vi "3_AdvancedDemo_MHT3.vi"() -> ()   [LabVIEW 2019]
uses:
  <userlib>/MultiHarp150/demos/Types/MH_InputChannel.ctl
  <userlib>/MultiHarp150/demos/Types/MH_UIThread_Cmds.ctl
  <userlib>/MultiHarp150/demos/Types/MH_UIThread_Data.ctl
  <userlib>/MultiHarp150/demos/_lib/PQ/MultiHarp/MH_InitInfo.ctl
  <userlib>/MultiHarp150/UIThread/MH_SetInpChanData.ctl
  <userlib>/MultiHarp150/UIThread/MH_SetInpChanCmds.ctl
  <userlib>/MultiHarp150/demos/Types/MH_DataProcThread_QData.ctl
  <userlib>/MultiHarp150/demos/Types/MH_DataProcThread_QCmds.ctl
  <userlib>/MultiHarp150/demos/Types/MH_VisThread_QData.ctl
  <userlib>/MultiHarp150/demos/Types/MH_VisThread_QCmds.ctl
  <userlib>/MultiHarp150/demos/Types/MH_VisThread_Data.ctl
  <userlib>/MultiHarp150/MH_RefSource.ctl
  <userlib>/MultiHarp150/MH_MeasMode.ctl
  <vilib>/Utility/error.llb/DialogType.ctl
  <userlib>/MultiHarp150/MH_LibVersion_global.vi
  <userlib>/MultiHarp150/MH_DllPath_global.vi
panel:
  in  "Settings":bool=TRUE
  in  "Run continuously":bool caption="Conti."
  in  "Start":bool
  in  "Scale":bool
  out "CountRates":i32[](graph)
  in  "AllChannels":T1={"Enable"=TRUE, "Offset"=0, "Level"=-100, "Edge"=0, "DeadTime"=1000, "UseDeadTime"=FALSE, "SetEnableAllChan"=TRUE, "SetEdgeAllChan"=TRUE, "SetLevelAllChan"=TRUE, "SetOffsetAllChan"=TRUE, "SetUseDTAllChan"=TRUE, "SetDeadTAllChan"=TRUE} {"DeadTime" min=800 max=160000 step=1; "Edge" items=["falling", "rising"]; "Offset" min=-100000 max=100000 step=5; "Level" min=-1200 max=1200 step=1}
  in  "HistoAcqTime":dbl=1.0 caption="Hist.Int.Time  s" min=0.1 max=360000.0 step=0.1
  in  "AcqTime":i32=360000000 caption="T3Acqu.       ms" min=1 max=360000 step=1
  in  "Binning":i32(ring) caption="Resol.            ps" items=["5", "10", "20", "40", "80", "160", "320", "640", "1280", "2560", "5120", "10240", "20480", "40960", "81920", "163840", "327680", "655360", "1310720", "2621440", "5242880", "10485760", "20971520", "41943040"]
  in  "HistoOffset":i32 caption="Offset            ns" min=0 max=100000000 step=1
  out "DeltaT":dbl=2.0479769602591973 caption="T.Tr.Resol.   ms" format="%.2f"
  in  "BitShift":i32=15 min=0 max=32 step=1
  in  "OvlLevel":u32=4294967295 caption="Ovl.Level" min=1024 max=65536 step=1024
  in  "StopOvl.":bool=TRUE
  out "TTraceGraph":T2(graph)={49.38852226226715, "Resolution"=0.00655367864414373, "Histogram"=[]}
  out "HistoGraph":cluster{dbl, "Resol":dbl, "Histos":u32[][]}(graph)={0.0, "Resol"=0.08, "Histos"=[]}
  in  "SyncDeadTime":i32=1000 caption="Dead T.   ps" min=800 max=160000 step=1
  in  "UseDeadTime":bool caption="Use DT."
  in  "SyncEdge":i32(ring) caption="Edge" items=["falling", "rising"]
  in  "SyncDivider":i32(ring) caption="Divider" items=["1", "2", "4", "8", "16"]
  in  "SyncOffset":i32 caption="Offset      ps" min=-100000 max=100000 step=5
  in  "SyncLevel":i32=-100 caption="Level      mV" min=-1200 max=1200 step=1
  in  "Channels":T3[](array[typedef])=[{"Name"="Inp.Chan 1", "Enable"=TRUE, "Edge"=0, "Level"=-100, "Offset"=0, "UseDeadTime"=FALSE, "DeadTime"=1000}, {"Name"="Inp.Chan 2", "Enable"=TRUE, "Edge"=0, "Level"=-100, "Offset"=0, "UseDeadTime"=FALSE, "DeadTime"=1000}, {"Name"="Inp.Chan 3", "Enable"=TRUE, "Edge"=0, "Level"=-100, "Offset"=0, "UseDeadTime"=FALSE, "DeadTime"=1000}, {"Name"="Inp.Chan 4", "Enable"=TRUE, "Edge"=0, "Level"=-100, "Offset"=0, "UseDeadTime"=FALSE, "DeadTime"=1000}, {"Name"="Inp.Chan 5", "Enable"=TRUE, "Edge"=0, "Level"=-100, "Offset"=0, "UseDeadTime"=FALSE, "DeadTime"=1000}, {"Name"="Inp.Chan 6", "Enable"=TRUE, "Edge"=0, "Level"=-100, "Offset"=0, "UseDeadTime"=FALSE, "DeadTime"=1000}, {"Name"="Inp.Chan 7", "Enable"=TRUE, "Edge"=0, "Level"=-100, "Offset"=0, "UseDeadTime"=FALSE, "DeadTime"=1000}, {"Name"="Inp.Chan 8", "Enable"=TRUE, "Edge"=0, "Level"=-100, "Offset"=0, "UseDeadTime"=FALSE, "DeadTime"=1000}, {"Name"="Inp.Chan 9", "Enable"=TRUE, "Edge"=0, "Level"=-100, "Offset"=0, "UseDeadTime"=FALSE, "DeadTime"=1000}, {"Name"="Inp.Chan 10", "Enable"=TRUE, "Edge"=0, "Level"=-100, "Offset"=0, "UseDeadTime"=FALSE, "DeadTime"=1000}, {"Name"="Inp.Chan 11", "Enable"=TRUE, "Edge"=0, "Level"=-100, "Offset"=0, "UseDeadTime"=FALSE, "DeadTime"=1000}, {"Name"="Inp.Chan 12", "Enable"=TRUE, "Edge"=0, "Level"=-100, "Offset"=0, "UseDeadTime"=FALSE, "DeadTime"=1000}, {"Name"="Inp.Chan 13", "Enable"=TRUE, "Edge"=0, "Level"=-100, "Offset"=0, "UseDeadTime"=FALSE, "DeadTime"=1000}, {"Name"="Inp.Chan 14", "Enable"=TRUE, "Edge"=0, "Level"=-100, "Offset"=0, "UseDeadTime"=FALSE, "DeadTime"=1000}, {"Name"="Inp.Chan 15", "Enable"=TRUE, "Edge"=0, "Level"=-100, "Offset"=0, "UseDeadTime"=FALSE, "DeadTime"=1000}, {"Name"="Inp.Chan 16", "Enable"=TRUE, "Edge"=0, "Level"=-100, "Offset"=0, "UseDeadTime"=FALSE, "DeadTime"=1000}, {"Name"="Inp.Chan 17", "Enable"=TRUE, "Edge"=0, "Level"=-100, "Offset"=0, "UseDeadTime"=FALSE, "DeadTime"=1000}, {"Name"="Inp.Chan 18", "Enable"=TRUE, "Edge"=0, "Level"=-100, "Offset"=0, "UseDeadTime"=FALSE, "DeadTime"=1000}, {"Name"="Inp.Chan 19", "Enable"=TRUE, "Edge"=0, "Level"=-100, "Offset"=0, "UseDeadTime"=FALSE, "DeadTime"=1000}, {"Name"="Inp.Chan 20", "Enable"=TRUE, "Edge"=0, "Level"=-100, "Offset"=0, "UseDeadTime"=FALSE, "DeadTime"=1000}, {"Name"="Inp.Chan 21", "Enable"=TRUE, "Edge"=0, "Level"=-100, "Offset"=0, "UseDeadTime"=FALSE, "DeadTime"=1000}, {"Name"="Inp.Chan 22", "Enable"=TRUE, "Edge"=0, "Level"=-100, "Offset"=0, "UseDeadTime"=FALSE, "DeadTime"=1000}, {"Name"="Inp.Chan 23", "Enable"=TRUE, "Edge"=0, "Level"=-100, "Offset"=0, "UseDeadTime"=FALSE, "DeadTime"=1000}, {"Name"="Inp.Chan 24", "Enable"=TRUE, "Edge"=0, "Level"=-100, "Offset"=0, "UseDeadTime"=FALSE, "DeadTime"=1000}, {"Name"="Inp.Chan 25", "Enable"=TRUE, "Edge"=0, "Level"=-100, "Offset"=0, "UseDeadTime"=FALSE, "DeadTime"=1000}, {"Name"="Inp.Chan 26", "Enable"=TRUE, "Edge"=0, "Level"=-100, "Offset"=0, "UseDeadTime"=FALSE, "DeadTime"=1000}, {"Name"="Inp.Chan 27", "Enable"=TRUE, "Edge"=0, "Level"=-100, "Offset"=0, "UseDeadTime"=FALSE, "DeadTime"=1000}, {"Name"="Inp.Chan 28", "Enable"=TRUE, "Edge"=0, "Level"=-100, "Offset"=0, "UseDeadTime"=FALSE, "DeadTime"=1000}, {"Name"="Inp.Chan 29", "Enable"=TRUE, "Edge"=0, "Level"=-100, "Offset"=0, "UseDeadTime"=FALSE, "DeadTime"=1000}, {"Name"="Inp.Chan 30", "Enable"=TRUE, "Edge"=0, "Level"=-100, "Offset"=0, "UseDeadTime"=FALSE, "DeadTime"=1000}, {"Name"="Inp.Chan 31", "Enable"=TRUE, "Edge"=0, "Level"=-100, "Offset"=0, "UseDeadTime"=FALSE, "DeadTime"=1000}, {"Name"="Inp.Chan 32", "Enable"=TRUE, "Edge"=0, "Level"=-100, "Offset"=0, "UseDeadTime"=FALSE, "DeadTime"=1000}, {"Name"="Inp.Chan 33", "Enable"=TRUE, "Edge"=0, "Level"=-100, "Offset"=0, "UseDeadTime"=FALSE, "DeadTime"=1000}, {"Name"="Inp.Chan 34", "Enable"=TRUE, "Edge"=0, "Level"=-100, "Offset"=0, "UseDeadTime"=FALSE, "DeadTime"=1000}, {"Name"="Inp.Chan 35", "Enable"=TRUE, "Edge"=0, "Level"=-100, "Offset"=0, "UseDeadTime"=FALSE, "DeadTime"=1000}, {"Name"="Inp.Chan 36", "Enable"=TRUE, "Edge"=0, "Level"=-100, "Offset"=0, "UseDeadTime"=FALSE, "DeadTime"=1000}, {"Name"="Inp.Chan 37", "Enable"=TRUE, "Edge"=0, "Level"=-100, "Offset"=0, "UseDeadTime"=FALSE, "DeadTime"=1000}, {"Name"="Inp.Chan 38", "Enable"=TRUE, "Edge"=0, "Level"=-100, "Offset"=0, "UseDeadTime"=FALSE, "DeadTime"=1000}, {"Name"="Inp.Chan 39", "Enable"=TRUE, "Edge"=0, "Level"=-100, "Offset"=0, "UseDeadTime"=FALSE, "DeadTime"=1000}, {"Name"="Inp.Chan 40", "Enable"=TRUE, "Edge"=0, "Level"=-100, "Offset"=0, "UseDeadTime"=FALSE, "DeadTime"=1000}, {"Name"="Inp.Chan 41", "Enable"=TRUE, "Edge"=0, "Level"=-100, "Offset"=0, "UseDeadTime"=FALSE, "DeadTime"=1000}, {"Name"="Inp.Chan 42", "Enable"=TRUE, "Edge"=0, "Level"=-100, "Offset"=0, "UseDeadTime"=FALSE, "DeadTime"=1000}, {"Name"="Inp.Chan 43", "Enable"=TRUE, "Edge"=0, "Level"=-100, "Offset"=0, "UseDeadTime"=FALSE, "DeadTime"=1000}, {"Name"="Inp.Chan 44", "Enable"=TRUE, "Edge"=0, "Level"=-100, "Offset"=0, "UseDeadTime"=FALSE, "DeadTime"=1000}, {"Name"="Inp.Chan 45", "Enable"=TRUE, "Edge"=0, "Level"=-100, "Offset"=0, "UseDeadTime"=FALSE, "DeadTime"=1000}, {"Name"="Inp.Chan 46", "Enable"=TRUE, "Edge"=0, "Level"=-100, "Offset"=0, "UseDeadTime"=FALSE, "DeadTime"=1000}, {"Name"="Inp.Chan 47", "Enable"=TRUE, "Edge"=0, "Level"=-100, "Offset"=0, "UseDeadTime"=FALSE, "DeadTime"=1000}, {"Name"="Inp.Chan 48", "Enable"=TRUE, "Edge"=0, "Level"=-100, "Offset"=0, "UseDeadTime"=FALSE, "DeadTime"=1000}, {"Name"="Inp.Chan 49", "Enable"=TRUE, "Edge"=0, "Level"=-100, "Offset"=0, "UseDeadTime"=FALSE, "DeadTime"=1000}, {"Name"="Inp.Chan 50", "Enable"=TRUE, "Edge"=0, "Level"=-100, "Offset"=0, "UseDeadTime"=FALSE, "DeadTime"=1000}, {"Name"="Inp.Chan 51", "Enable"=TRUE, "Edge"=0, "Level"=-100, "Offset"=0, "UseDeadTime"=FALSE, "DeadTime"=1000}, {"Name"="Inp.Chan 52", "Enable"=TRUE, "Edge"=0, "Level"=-100, "Offset"=0, "UseDeadTime"=FALSE, "DeadTime"=1000}, {"Name"="Inp.Chan 53", "Enable"=TRUE, "Edge"=0, "Level"=-100, "Offset"=0, "UseDeadTime"=FALSE, "DeadTime"=1000}, {"Name"="Inp.Chan 54", "Enable"=TRUE, "Edge"=0, "Level"=-100, "Offset"=0, "UseDeadTime"=FALSE, "DeadTime"=1000}, {"Name"="Inp.Chan 55", "Enable"=TRUE, "Edge"=0, "Level"=-100, "Offset"=0, "UseDeadTime"=FALSE, "DeadTime"=1000}, {"Name"="Inp.Chan 56", "Enable"=TRUE, "Edge"=0, "Level"=-100, "Offset"=0, "UseDeadTime"=FALSE, "DeadTime"=1000}, {"Name"="Inp.Chan 57", "Enable"=TRUE, "Edge"=0, "Level"=-100, "Offset"=0, "UseDeadTime"=FALSE, "DeadTime"=1000}, {"Name"="Inp.Chan 58", "Enable"=TRUE, "Edge"=0, "Level"=-100, "Offset"=0, "UseDeadTime"=FALSE, "DeadTime"=1000}, {"Name"="Inp.Chan 59", "Enable"=TRUE, "Edge"=0, "Level"=-100, "Offset"=0, "UseDeadTime"=FALSE, "DeadTime"=1000}, {"Name"="Inp.Chan 60", "Enable"=TRUE, "Edge"=0, "Level"=-100, "Offset"=0, "UseDeadTime"=FALSE, "DeadTime"=1000}, {"Name"="Inp.Chan 61", "Enable"=TRUE, "Edge"=0, "Level"=-100, "Offset"=0, "UseDeadTime"=FALSE, "DeadTime"=1000}, {"Name"="Inp.Chan 62", "Enable"=TRUE, "Edge"=0, "Level"=-100, "Offset"=0, "UseDeadTime"=FALSE, "DeadTime"=1000}, {"Name"="Inp.Chan 63", "Enable"=TRUE, "Edge"=0, "Level"=-100, "Offset"=0, "UseDeadTime"=FALSE, "DeadTime"=1000}, {"Name"="Inp.Chan 64", "Enable"=TRUE, "Edge"=0, "Level"=-100, "Offset"=0, "UseDeadTime"=FALSE, "DeadTime"=1000}] {"DeadTime" min=800 max=160000 step=1; "Edge" items=["falling", "rising"]; "Offset" min=-100000 max=100000 step=5; "Level" min=-1200 max=1200 step=1}
  out "SyncRate":string="Sync Rate: 16000190 cps\n"
  out "OverRun":bool caption="Overrun:"
  out "Status":string="Elements in Q: 0"
  # "All Channels"
  # "Acquisition"
  # "Sync"
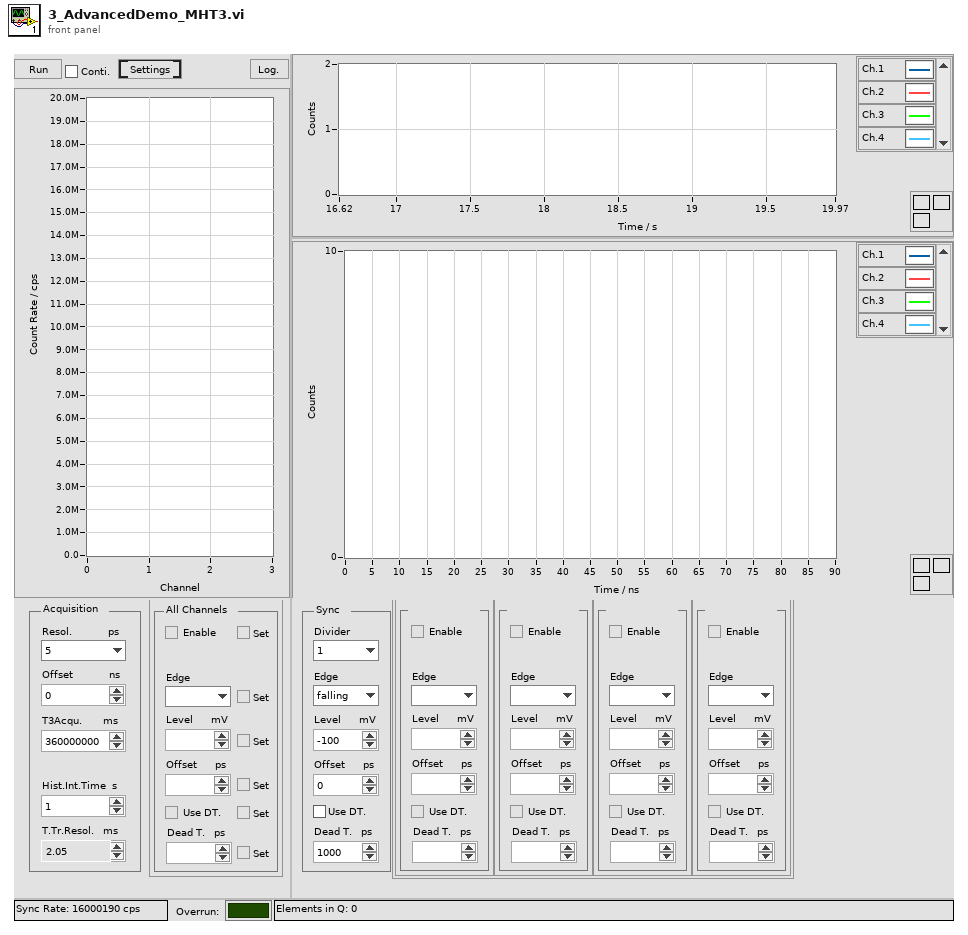
[diagram p1: front panel]
types:
  T1 = cluster{"Enable":bool, "Offset":i32, "Level":i32, "Edge":i32, "DeadTime":i32, "UseDeadTime":bool, "SetEnableAllChan":bool, "SetEdgeAllChan":bool, "SetLevelAllChan":bool, "SetOffsetAllChan":bool, "SetUseDTAllChan":bool, "SetDeadTAllChan":bool}
  T2 = cluster{dbl, "Resolution":dbl, "Histogram":u32[][]}
  T3 = typedef "MH_InputChannel.ctl" = cluster{"Name":string, "Enable":bool, "Edge":i32, "Level":i32, "Offset":i32, "UseDeadTime":bool, "DeadTime":i32}
  T4 = typedef "MH_DataProcThread_QCmds.ctl" = enum16{"Exit", "Proc", "Init", "SetShift", "SetNumChannels", "SetHistAcqTime"}
  T5 = typedef "MH_VisThread_Data.ctl" = cluster{"Resol":dbl, "DeltaT":dbl, "NumChannels":i32}
  T6 = typedef "MH_VisThread_QData.ctl" = cluster{"Histos":u32[][], "Cmd":T7, "TimeTrace":u32[][], "Bin":i32, "Total bin":u64, "Status":string, "Resol":dbl, "DeltaT":dbl, "nChannels":i32}
  T7 = typedef "MH_VisThread_QCmds.ctl" = enum16{"_none_", "Resol", "nChannels", "DeltaT", "Histo", "TTrace", "Status"}
  T8 = typedef "MH_DataProcThread_QData.ctl" = cluster{"Cmd":T4, "nActual":i32, "Buffer":u32[], "TickCount":u32, "Param":i32}
  T9 = typedef "MH_UIThread_Data.ctl" = cluster{"Init Info":T10, "DevIdx":i32, "SyncDivider":i32, "SyncOffset":i32, "SyncLevel":i32, "Channels":T3[], "CurrentChannels":i32[], "AcqTime":i32, "Binning":i32, "HistoOffset":i32, "HistoLen":i32, "StopOvl.":bool, "OvlLevel":u32, "SyncEdge":i32, "StartMeas":bool, "HistoLength":i32, "Resolution":dbl, "Run cont.":bool, "Status":string, "SyncRate":i32, "BitShift":i32, "HistoAcqTime":dbl, "SyncRateStart":i32, "UseDeadTime":bool, "SyncDeadTime":i32, "SetInpChan":T11[]}
  T10 = typedef "MH_InitInfo.ctl" = cluster{"Library Version":string, "Serial No.":string, "Model":string, "Partnum":string, "Version":string, "features":i32, "nchannels":i32, "Base Resolution":dbl, "Bin Steps":i32}
  T11 = typedef "MH_SetInpChanData.ctl" = cluster{"Channel":i32, "Cmds":T12[], "Changed":cluster{"Name":bool, "Enable":bool, "Edge":bool, "Level":bool, "Offset":bool, "UseDeadTime":bool, "DeadTime":bool}}
  T12 = typedef "MH_SetInpChanCmds.ctl" = enum16{"SetInpChanEnable", "SetInpChanOffset", "SetInpChanDeadTime", "SetInpChanTrg"}
  T13 = typedef "MH_UIThread_Cmds.ctl" = enum16{"Idle", "Init", "SetInpChan", "SetSyncDivider", "SetSyncTrg", "SetSyncOffset", "SetSyncDeadTime", "SetBinning", "SetHistoOffset", "SetHistoLen", "SetStopOvl", "SetBitShift", "SetHistoAcqTime", "GetRates", "GetAllRates", "StartMeas", "StopMeas", "AbortMeas", "GetResolution", "GetHistos", "GetAllHistos", "ReadFiFo", "WriteStatus", "Resize", "EnableControls", "DisableControls", "Error", "Exit"}
  T14 = enum8{"Enabled", "Disabled", "Disabled and Grayed Out"}
  T15 = typedef "MH_InputChannel_LS.ctl" = cluster{"Name":string, "Enable":bool, "Edge":i32, "Level":i32, "Offset":i32, "UseDeadTime":bool, "DeadTime":i32}
  T16 = cluster{"[0]":bool, "[1]":bool, "[2]":bool, "[3]":bool, "[4]":bool, "[5]":bool}
  T17 = typedef "MH_MeasMode.ctl" = i32
  T18 = typedef "MH_RefSource.ctl" = enum16{"INTERNAL", "EXTERNAL_10MHZ", "WR_MASTER_GENERIC", "WR_SLAVE_GENERIC", "WR_GRANDM_GENERIC", "EXTN_GPS_PPS", "EXTN_GPS_PPS_UART", "WR_MASTER_MHARP", "WR_SLAVE_MHARP", "WR_GRANDM_MHARP"}
  T19 = typedef "DialogType.ctl" = u16
  T20 = cluster{"T0":dbl, "dt":dbl, "TimeTrace_out":u32[][]}
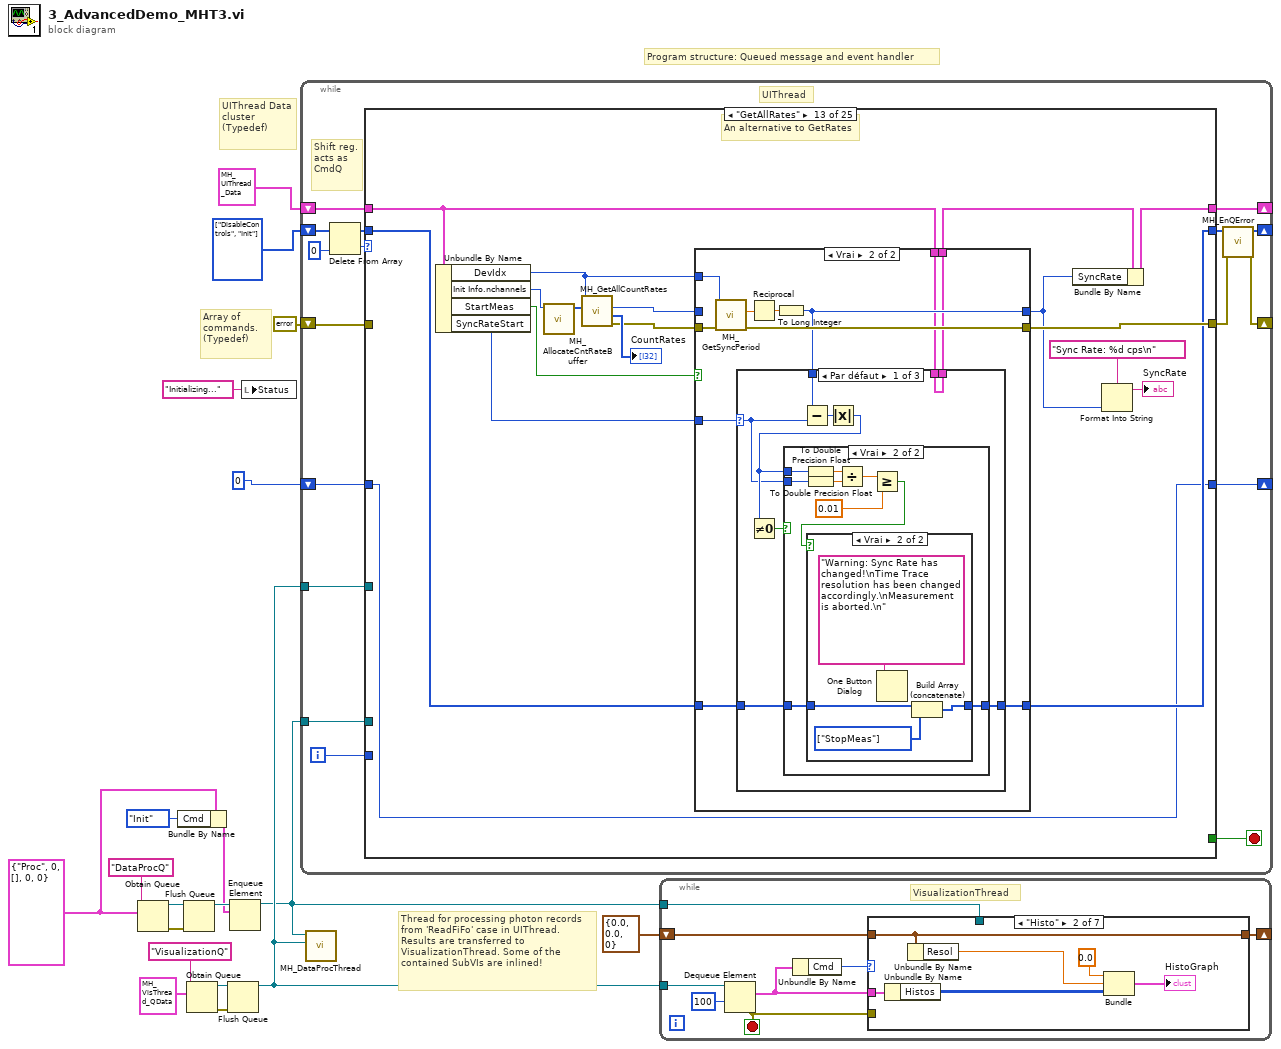
[diagram p0: block diagram]
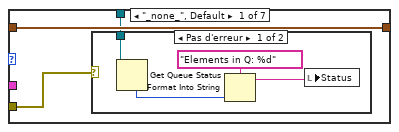
[diagram p2: hidden frame]
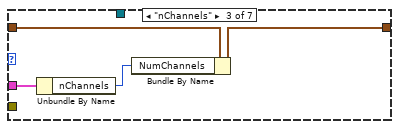
[diagram p4: hidden frame]
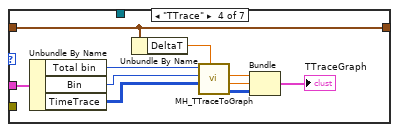
[diagram p5: hidden frame]
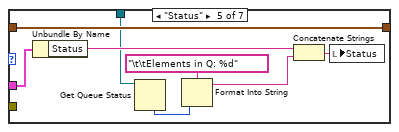
[diagram p6: hidden frame]
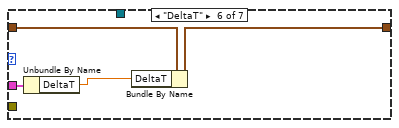
[diagram p7: hidden frame]
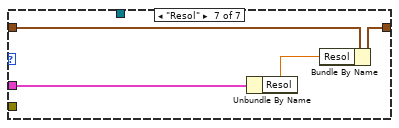
[diagram p8: hidden frame]
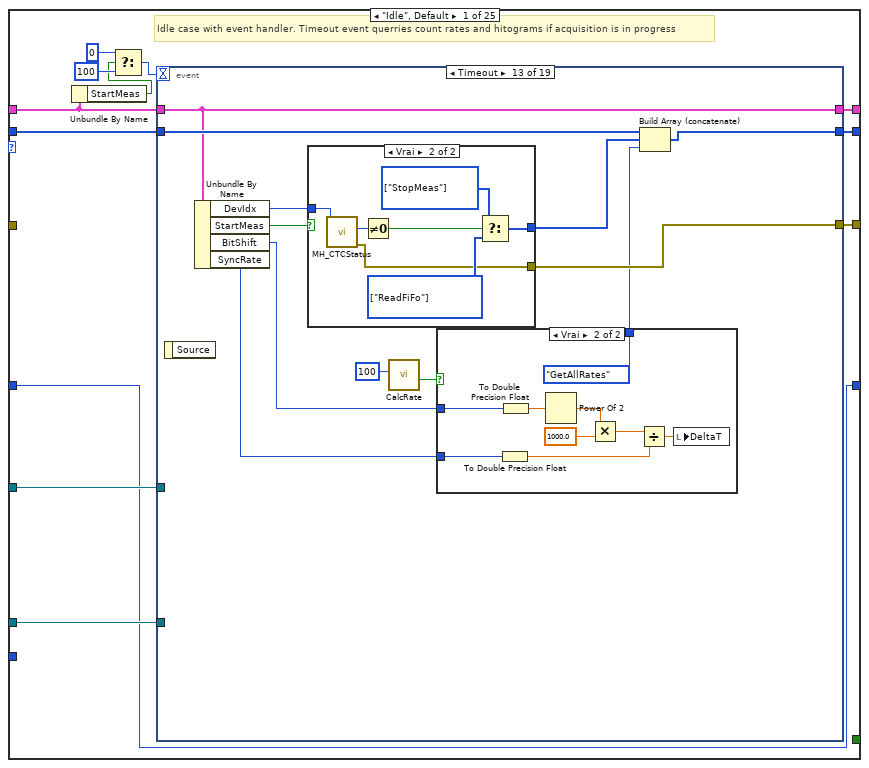
[diagram p9: hidden frame]
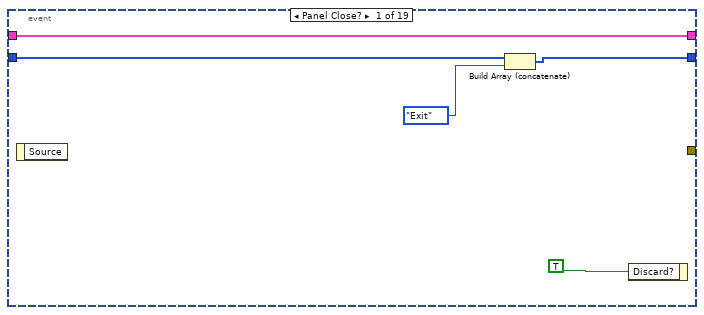
[diagram p10: hidden frame]
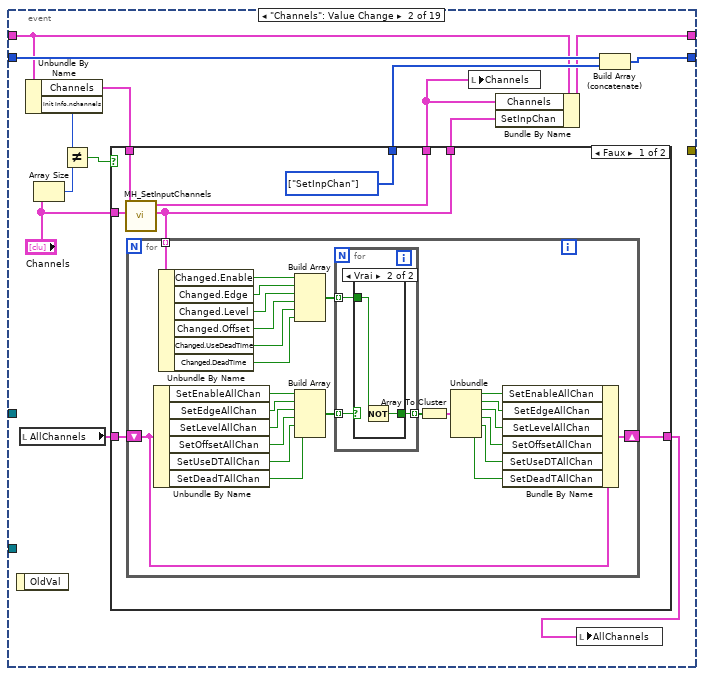
[diagram p11: hidden frame]
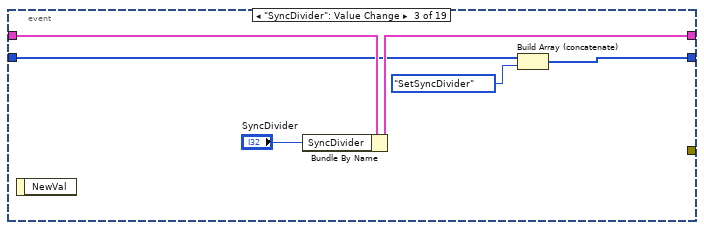
[diagram p14: hidden frame]
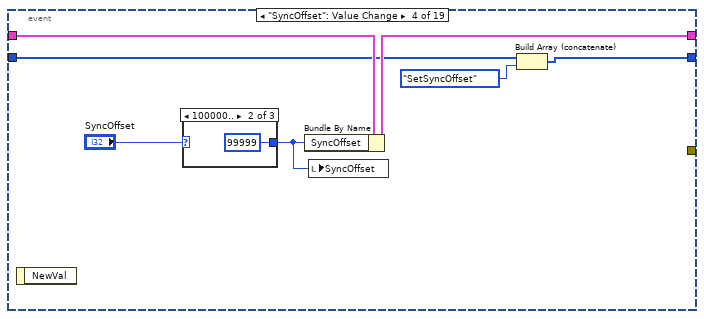
[diagram p15: hidden frame]
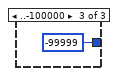
[diagram p17: hidden frame]
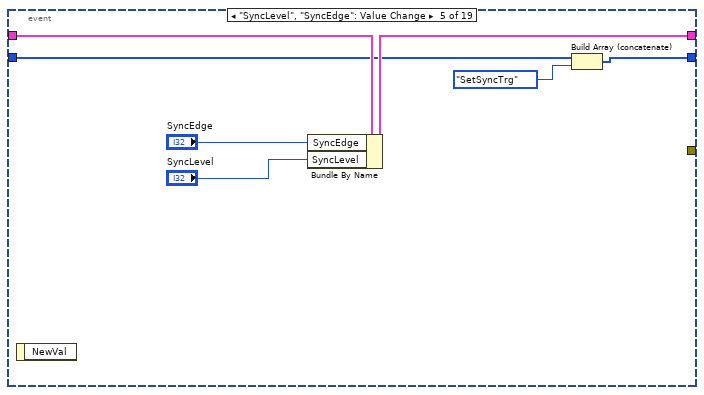
[diagram p18: hidden frame]
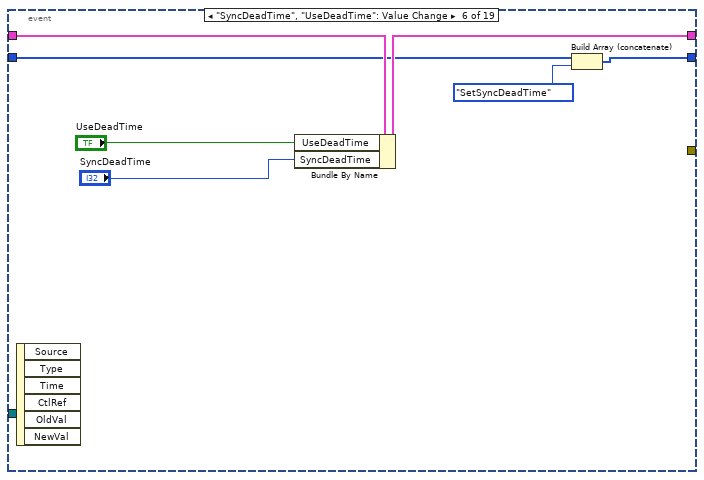
[diagram p19: hidden frame]
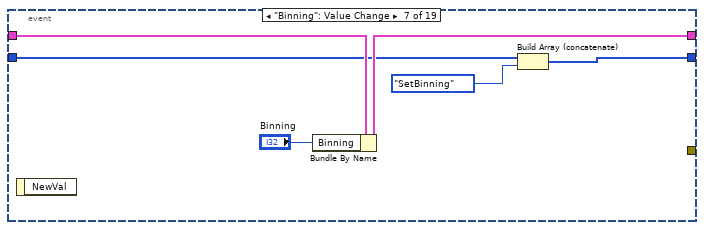
[diagram p20: hidden frame]
diagram:
  w5 = T8 {"Cmd"=enum."Proc", "nActual"=0, "Buffer"=[], "TickCount"=0, "Param"=0} ("MH_DataProcThread_QData")
  w18 = T13[] [enum."DisableControls", enum."Init"] items=["Idle", "Init", "SetInpChan", "SetSyncDivider", "SetSyncTrg", "SetSyncOffset", "SetSyncDeadTime", "SetBinning", "SetHistoOffset", "SetHistoLen", "SetStopOvl", "SetBitShift", "SetHistoAcqTime", "GetRates", "GetAllRates", "StartMeas", "StopMeas", "AbortMeas", "GetResolution", "GetHistos", "GetAllHistos", "ReadFiFo", "WriteStatus", "Resize", "EnableControls", "DisableControls", "Error", "Exit"]
  # "Thread for processing photon records from 'ReadFiFo' case in UIThread. Results are transferred to VisualizationThread. Some of the contained SubVIs are inlined!"
  # "Array of commands.\n(Typedef)"
  # "Program structure: Queued message and event handler"
  # "UIThread Data cluster\n(Typedef)"
  n1 = Obtain Queue(name (unnamed)="DataProcQ", element data type=w5) -> (queue out=w15:refnum<queue>, error out=w14:errorcluster)  [unwired: 3 in, 1 out]
  n2 = Bundle By Name(cluster=w5, "Cmd"=MH_DataProcThread_QCmds."Init") -> (w3:T8)
  n3 = Flush Queue(queue=w15, error in (no error)=w14) -> (queue out=w6:refnum<queue>)  [unwired: 2 out]
  n4 = Obtain Queue(name (unnamed)="VisualizationQ", element data type=T6 {"Histos"=[], "Cmd"=enum."_none_", "TimeTrace"=[], "Bin"=0, "Total bin"=0, "Status"="", "Resol"=0.0, "DeltaT"=0.0, "nChannels"=0} ("MH_GUIThread_QData")) -> (queue out=w13:refnum<queue>, error out=w12:errorcluster)  [unwired: 3 in, 1 out]
  n5 = Flush Queue(queue=w13, error in (no error)=w12) -> (queue out=w8:refnum<queue>)  [unwired: 2 out]
  n6 = Enqueue Element(queue=w6, element=w3) -> (queue out=w2:refnum<queue>)  [unwired: 2 in, 2 out]
  n7 = local write "Status"("Initializing..." ("Status")) -> ()
  n8 = while {
    shift-right: [w25] -> _
    shift-left: w18 -> [w32]
    shift-right: [w35] -> _
    shift-left: T9 {"Init Info"={"Library Version"="", "Serial No."="", "Model"="", "Partnum"="", "Version"="", "features"=0, "nchannels"=0, "Base Resolution"=0.0, "Bin Steps"=0}, "DevIdx"=0, "SyncDivider"=1, "SyncOffset"=0, "SyncLevel"=50, "Channels"=[], "CurrentChannels"=[], "AcqTime"=1, "Binning"=1, "HistoOffset"=1, "HistoLen"=1024, "StopOvl."=FALSE, "OvlLevel"=1024, "SyncEdge"=10, "StartMeas"=FALSE, "HistoLength"=0, "Resolution"=0.0, "Run cont."=FALSE, "Status"="", "SyncRate"=0, "BitShift"=0, "HistoAcqTime"=0.0, "SyncRateStart"=0, "UseDeadTime"=FALSE, "SyncDeadTime"=800, "SetInpChan"=[]} -> [w34]
    shift-right: [w27] -> _
    shift-left: errorcluster {"status"=FALSE, "code"=0, "source"=""} ("error IO") -> [w33]
    tunnel: w2 -> [w24]
    tunnel: w8 -> [w23]
    shift-right: [w20] -> _
    shift-left: 0 -> [w21]
    i -> [w22]
    stop <- w36 stop-if-true
    # "Shift reg.\nacts as\nCmdQ"
    # "UIThread"
    n9 = Delete From Array(array=w32, index=0) -> (deleted portion=w30:T13, array with subset deleted=w29:T13[])  [unwired: 1 in]
    n10 = case shown="\"GetAllRates\"" w30 {
      tunnel: [w48 w365 w384 w447 w457 w470 w477 w485 w494 w502 w523 w536 w540 w613 w637 w643 w657 w675 w678 w708 w722 w730 w743 w750 w757] -> w26
      tunnel: [_ _ _ _ _ _ _ _ _ _ _ _ _ _ _ _ _ _ _ _ _ _ _ _ TRUE] -> w36
      tunnel: [w47 w346 w385 w449 w458 w471 w481 w489 w495 w503 w508 w526 w549 w605 w629 w646 w659 w671 w688 w707 w710 w729 w742 w751 w760] -> w35
      tunnel: w34 -> [w44 w351 w385 w449 w458 w471 w481 w489 w495 w503 w508 w526 w539 w606 w630 w647 w660 w672 w688 w707 w710 w729 w742 w751 w760]
      tunnel: [w45 w368 w379 w445 w456 w469 w480 w488 w493 w501 _ _ w545 w612 w640 w649 w662 w673 w683 _ _ _ _ _ w758] -> w28
      tunnel: w33 -> [_ _ _ _ _ _ _ _ _ _ _ _ _ _ _ _ _ _ _ _ _ _ _ w752 _]
      tunnel: w29 -> [w46 w367 w384 w447 w457 w470 w477 w484 w494 w502 w523 w536 w541 w613 w638 w644 w657 w675 w679 w708 w722 w730 w743 _ w757]
      tunnel: w24 -> [w39 w344 _ _ _ _ _ _ _ _ w509 w527 _ _ w634 _ _ _ w680 _ _ _ _ _ w756]
      tunnel: w23 -> [w38 w337 _ _ _ _ _ _ _ _ w510 _ _ _ _ _ _ w668 _ _ _ _ _ _ w755]
      tunnel: w22 -> [_ _ _ _ _ _ _ _ _ _ _ _ _ _ _ _ _ _ _ _ _ _ _ _ _]
      tunnel: w21 -> [w37 w313 w377 w441 w452 w459 w476 w482 w490 w496 w504 w524 w537 w601 w627 w641 w656 w663 w677 w705 w709 w723 w736 w749 w754]
      tunnel: [w37 w313 w377 w441 w452 w459 w476 w482 w490 w496 w504 w524 w537 w601 w627 w641 w656 w663 w676 w705 w709 w723 w736 w749 w754] -> w20
      frame "Idle", Default {
        # "Idle case with event handler. Timeout event querries count rates and hitograms if acquisition is in progress"
        n11 = Unbundle By Name(w44) -> ("StartMeas"=w42:bool)
        n12 = Select(t=0, s=w42, f=100) -> (s? t:f=w41:i32)
        n13 = event shown="[12] Timeout" {
          selector: _ -> [_ _ _ _ _ _ _ _ _ _ _ _ _ _ _ _ _ _ _]
          dyn-events: _ -> [_ _ _ _ _ _ _ _ _ _ _ _ _ _ _ _ _ _ _]
          timeout: w41 -> [_ _ _ _ _ _ _ _ _ _ _ _ _ _ _ _ _ _ _]
          tunnel: [w49 w66 w108 w116 w125 w133 w139 w145 w150 w210 w215 w222 w237 w255 w267 w285 w291 w299 w309] -> w48
          tunnel: [w52 w58 w112 w119 w129 w136 w142 w148 w155 w212 w218 w225 w236 w259 w266 w283 w290 w298 w312] -> w47
          tunnel: w44 -> [w52 w59 w113 w120 w130 w137 w143 w149 w156 w213 w219 w226 w236 w260 w264 w284 w290 w298 w312]
          tunnel: w46 -> [w51 w67 w110 w118 w127 w135 w141 w147 w151 w210 w216 w224 w238 w256 w268 w285 w291 w299 w310]
          tunnel: [_ _ _ _ _ _ _ _ _ _ _ _ w232 _ _ _ _ _ _] -> w45
          tunnel: w39 -> [_ _ _ _ _ _ _ _ _ _ _ _ _ _ _ _ _ _ _]
          tunnel: w38 -> [_ _ _ _ _ _ _ _ _ _ _ _ _ _ _ _ _ _ _]
          event Panel Close? {
            n14 = event-data() -> ()  [unwired: 1 in, 1 out]
            n15 = Build Array (concatenate)(w51, MH_UIThread_Cmds."Exit") -> (w49:T13[])
            n16 = event-data("Discard?"=TRUE) -> ()  [unwired: 1 in, 1 out]
          }
          event "Channels": Value Change {
            n17 = event-data() -> ()  [unwired: 1 in, 1 out]
            n18 = local read "AllChannels"() -> (w54:T1)
            n19 = Unbundle By Name(w59) -> ("Channels"=w61:T3[], "Init Info.nchannels"=w63:i32)
            n20 = Array Size(array="Channels") -> (size(s)=w64:i32)
            n21 = Not Equal?(x=w63, y=w64) -> (x != y?=w62:bool)
            n22 = case shown="Faux" w62 {
              tunnel: "Channels" -> [w73 _]
              tunnel: [w72 w107] -> w56
              tunnel: w61 -> [w74 w107]
              tunnel: [w70 _] -> w57
              tunnel: [w71 _] -> w60
              tunnel: w54 -> [w69 w106]
              tunnel: [w68 w106] -> w55
              frame False {
                w71 = T13[] [enum."SetInpChan"] items=["Idle", "Init", "SetInpChan", "SetSyncDivider", "SetSyncTrg", "SetSyncOffset", "SetSyncDeadTime", "SetBinning", "SetHistoOffset", "SetHistoLen", "SetStopOvl", "SetBitShift", "SetHistoAcqTime", "GetRates", "GetAllRates", "StartMeas", "StopMeas", "AbortMeas", "GetResolution", "GetHistos", "GetAllHistos", "ReadFiFo", "WriteStatus", "Resize", "EnableControls", "DisableControls", "Error", "Exit"] ("array")
                n23 = call <userlib>:"MH_SetInputChannels.vi"("Channels new"=w73, "Channels old"=w74) -> ("SetInpChan"=w70:T11[], "Channels"=w72:T15[])  [unwired: 7 in, 1 out]
                n24 = for {
                  tunnel: w70 -> [w99] mode=indexing
                  shift-right: [w81] -> w68
                  shift-left: w69 -> [w83]
                  n25 = Unbundle By Name(w83) -> ("SetEnableAllChan"=w92:bool, "SetEdgeAllChan"=w91:bool, "SetLevelAllChan"=w90:bool, "SetOffsetAllChan"=w89:bool, "SetUseDTAllChan"=w88:bool, "SetDeadTAllChan"=w87:bool)
                  n26 = Unbundle By Name(w99) -> ("Changed.Enable"=w98:bool, "Changed.Edge"=w97:bool, "Changed.Level"=w96:bool, "Changed.Offset"=w95:bool, "Changed.UseDeadTime"=w94:bool, "Changed.DeadTime"=w93:bool)
                  n27 = Build Array(w98, w97, w96, w95, w94, w93) -> (w85:bool[])
                  n28 = Build Array(w92, w91, w90, w89, w88, w87) -> (w86:bool[])
                  n29 = for {
                    tunnel: w86 -> [w102] mode=indexing
                    tunnel: w85 -> [w100] mode=indexing
                    tunnel: [w101] -> w84 mode=indexing
                    n30 = case shown="Vrai" w102 {
                      selector: w102 -> [w103 _]
                      tunnel: [w103 w104] -> w101
                      tunnel: w100 -> [_ w105]
                      frame False {
                      }
                      frame True {
                        n31 = Not(x=w105) -> (.not. x?=w104:bool)
                      }
                    }
                  }
                  n32 = Array To Cluster(array=w84) -> (cluster=w82:T16)
                  n33 = Unbundle(w82) -> ("[0]"=w80:bool, "[1]"=w79:bool, "[2]"=w78:bool, "[3]"=w77:bool, "[4]"=w76:bool, "[5]"=w75:bool)
                  n34 = Bundle By Name(cluster=w83, "SetEnableAllChan"=w80, "SetEdgeAllChan"=w79, "SetLevelAllChan"=w78, "SetOffsetAllChan"=w77, "SetUseDTAllChan"=w76, "SetDeadTAllChan"=w75) -> (w81:T1)
                }
              }
              frame True {
              }
            }
            n35 = local write "Channels"(w56) -> ()
            n36 = Bundle By Name(cluster=w59, "Channels"=w56, "SetInpChan"=w57) -> (w58:T9)
            n37 = local write "AllChannels"(w55) -> ()
            n38 = Build Array (concatenate)(w67, w60) -> (w66:T13[])
          }
          event "SyncDivider": Value Change {
            n39 = event-data() -> ()  [unwired: 1 in, 1 out]
            n40 = Bundle By Name(cluster=w113, "SyncDivider"="SyncDivider") -> (w112:T9)
            n41 = Build Array (concatenate)(w110, MH_UIThread_Cmds."SetSyncDivider") -> (w108:T13[])
          }
          event "SyncOffset": Value Change {
            n42 = event-data() -> ()  [unwired: 1 in, 1 out]
            n43 = case shown="100000.." "SyncOffset" {
              selector: "SyncOffset" -> [w121 _ _]
              tunnel: [w121 99999 ("SyncOffset") -99999 ("SyncOffset")] -> w114
              frame Default {
              }
              frame 100000.. {
              }
              frame ..-100000 {
              }
            }
            n44 = Bundle By Name(cluster=w120, "SyncOffset"=w114) -> (w119:T9)
            n45 = local write "SyncOffset"(w114) -> ()
            n46 = Build Array (concatenate)(w118, MH_UIThread_Cmds."SetSyncOffset") -> (w116:T13[])
          }
          event "SyncLevel", "SyncEdge": Value Change {
            n47 = event-data() -> ()  [unwired: 1 in, 1 out]
            n48 = Bundle By Name(cluster=w130, "SyncEdge"="SyncEdge", "SyncLevel"="SyncLevel") -> (w129:T9)
            n49 = Build Array (concatenate)(w127, MH_UIThread_Cmds."SetSyncTrg") -> (w125:T13[])
          }
          event "SyncDeadTime", "UseDeadTime": Value Change {
            n50 = event-data() -> ()  [unwired: 1 in, 6 out]
            n51 = Bundle By Name(cluster=w137, "UseDeadTime"="UseDeadTime", "SyncDeadTime"="SyncDeadTime") -> (w136:T9)
            n52 = Build Array (concatenate)(w135, MH_UIThread_Cmds."SetSyncDeadTime") -> (w133:T13[])
          }
          event "Binning": Value Change {
            n53 = event-data() -> ()  [unwired: 1 in, 1 out]
            n54 = Bundle By Name(cluster=w143, "Binning"="Binning") -> (w142:T9)
            n55 = Build Array (concatenate)(w141, MH_UIThread_Cmds."SetBinning") -> (w139:T13[])
          }
          event "HistoOffset": Value Change {
            n56 = event-data() -> ()  [unwired: 1 in, 1 out]
            n57 = Bundle By Name(cluster=w149, "HistoOffset"="HistoOffset") -> (w148:T9)
            n58 = Build Array (concatenate)(w147, MH_UIThread_Cmds."SetHistoOffset") -> (w145:T13[])
          }
          event "AllChannels": Value Change {
            w152 = T13[] [enum."SetInpChan"] items=["Idle", "Init", "SetInpChan", "SetSyncDivider", "SetSyncTrg", "SetSyncOffset", "SetSyncDeadTime", "SetBinning", "SetHistoOffset", "SetHistoLen", "SetStopOvl", "SetBitShift", "SetHistoAcqTime", "GetRates", "GetAllRates", "StartMeas", "StopMeas", "AbortMeas", "GetResolution", "GetHistos", "GetAllHistos", "ReadFiFo", "WriteStatus", "Resize", "EnableControls", "DisableControls", "Error", "Exit"] ("array")
            n59 = event-data() -> ()  [unwired: 1 in, 1 out]
            n60 = local read "Channels"() -> (w159:T3[])
            n61 = for {
              tunnel: w159 -> [w163] mode=indexing
              tunnel: "AllChannels" -> [w162]
              tunnel: [w161] -> w158 mode=indexing
              n62 = Unbundle By Name(w162) -> ("SetEnableAllChan"=w164:bool, "SetEdgeAllChan"=w165:bool, "SetLevelAllChan"=w166:bool, "SetOffsetAllChan"=w167:bool, "SetUseDTAllChan"=w168:bool, "SetDeadTAllChan"=w169:bool)
              n63 = Build Array(w164, w165, w166, w167, w168, w169) -> (w170:bool[])
              n64 = for {
                tunnel: w170 -> [w175] mode=indexing
                shift-right: [w172] -> w161
                shift-left: w163 -> [w173]
                tunnel: w162 -> [w171]
                i -> [w174]
                n65 = case shown="Vrai" w175 {
                  tunnel: w174 -> [_ w180]
                  tunnel: w171 -> [_ w179]
                  tunnel: w173 -> [w176 w178]
                  tunnel: [w176 w177] -> w172
                  frame False {
                  }
                  frame True {
                    n66 = case shown="3" w180 {
                      tunnel: w179 -> [w184 w188 w192 w197 w204 w208 _]
                      tunnel: w178 -> [w183 w187 w191 w196 w203 w207 w209]
                      tunnel: [w181 w185 w189 w195 w201 w205 w209] -> w177
                      frame 0 {
                        n67 = Unbundle By Name(w184) -> ("Enable"=w182:bool)
                        n68 = Bundle By Name(cluster=w183, "Enable"=w182) -> (w181:T3)
                      }
                      frame 1 {
                        n69 = Unbundle By Name(w188) -> ("Edge"=w186:i32)
                        n70 = Bundle By Name(cluster=w187, "Edge"=w186) -> (w185:T3)
                      }
                      frame 2 {
                        n71 = Unbundle By Name(w192) -> ("Level"=w190:i32)
                        n72 = Bundle By Name(cluster=w191, "Level"=w190) -> (w189:T3)
                      }
                      frame 3 {
                        n73 = Unbundle By Name(w197) -> ("Offset"=w194:i32)
                        n74 = case shown="100000.." w194 {
                          selector: w194 -> [w198 _ _]
                          tunnel: [w198 99999 ("SyncOffset") -99999 ("SyncOffset")] -> w193
                          frame Default {
                          }
                          frame 100000.. {
                          }
                          frame ..-100000 {
                          }
                        }
                        n75 = Bundle By Name(cluster=w196, "Offset"=w193) -> (w195:T3)
                      }
                      frame 4 {
                        n76 = Unbundle By Name(w204) -> ("UseDeadTime"=w202:bool)
                        n77 = Bundle By Name(cluster=w203, "UseDeadTime"=w202) -> (w201:T3)
                      }
                      frame 5 {
                        n78 = Unbundle By Name(w208) -> ("DeadTime"=w206:i32)
                        n79 = Bundle By Name(cluster=w207, "DeadTime"=w206) -> (w205:T3)
                      }
                      frame Default {
                      }
                    }
                  }
                }
              }
            }
            n80 = Build Array (concatenate)(w151, w152) -> (w150:T13[])
            n81 = Unbundle By Name(w156) -> ("Channels"=w157:T3[])
            n82 = call <userlib>:"MH_SetInputChannels.vi"("Channels new"=w158, "Channels old"=w157) -> ("SetInpChan"=w153:T11[], "Channels"=w154:T15[])  [unwired: 7 in, 1 out]
            n83 = local write "Channels"(w154) -> ()
            n84 = Bundle By Name(cluster=w156, "Channels"=w154, "SetInpChan"=w153) -> (w155:T9)
          }
          event "AcqTime": Value Change {
            n85 = event-data() -> ()  [unwired: 1 in, 1 out]
            n86 = Bundle By Name(cluster=w213, "AcqTime"="AcqTime") -> (w212:T9)
          }
          event "HistoAcqTime": Value Change {
            n87 = event-data() -> ()  [unwired: 1 in, 1 out]
            n88 = Bundle By Name(cluster=w219, "HistoAcqTime"="HistoAcqTime") -> (w218:T9)
            n89 = Build Array (concatenate)(w216, MH_UIThread_Cmds."SetHistoAcqTime") -> (w215:T13[])
          }
          event "OvlLevel", "StopOvl.": Value Change {
            n90 = event-data() -> ()  [unwired: 1 in, 1 out]
            n91 = Bundle By Name(cluster=w226, "StopOvl."="StopOvl.", "OvlLevel"="OvlLevel") -> (w225:T9)
            n92 = Build Array (concatenate)(w224, MH_UIThread_Cmds."SetStopOvl") -> (w222:T13[])
          }
          event Timeout {
            n93 = event-data() -> ()  [unwired: 1 in, 1 out]
            n94 = Unbundle By Name(w236) -> ("DevIdx"=w234:i32, "StartMeas"=w235:bool, "BitShift"=w231:i32, "SyncRate"=w230:i32)
            n95 = case shown="Vrai" w235 {
              tunnel: w234 -> [_ w254]
              tunnel: [_ w252] -> w233
              tunnel: [_ w249] -> w232
              frame False {
              }
              frame True {
                w250 = T13[] [enum."ReadFiFo"] items=["Idle", "Init", "SetInpChan", "SetSyncDivider", "SetSyncTrg", "SetSyncOffset", "SetSyncDeadTime", "SetBinning", "SetHistoOffset", "SetHistoLen", "SetStopOvl", "SetBitShift", "SetHistoAcqTime", "GetRates", "GetAllRates", "StartMeas", "StopMeas", "AbortMeas", "GetResolution", "GetHistos", "GetAllHistos", "ReadFiFo", "WriteStatus", "Resize", "EnableControls", "DisableControls", "Error", "Exit"]
                w251 = T13[] [enum."StopMeas"] items=["Idle", "Init", "SetInpChan", "SetSyncDivider", "SetSyncTrg", "SetSyncOffset", "SetSyncDeadTime", "SetBinning", "SetHistoOffset", "SetHistoLen", "SetStopOvl", "SetBitShift", "SetHistoAcqTime", "GetRates", "GetAllRates", "StartMeas", "StopMeas", "AbortMeas", "GetResolution", "GetHistos", "GetAllHistos", "ReadFiFo", "WriteStatus", "Resize", "EnableControls", "DisableControls", "Error", "Exit"]
                n96 = call <userlib>:"MH_CTCStatus.vi"("devidx"=w254) -> ("error out"=w249:errorcluster, "ctcstatus"=w253:i32)  [unwired: 8 in, 1 out]
                n97 = Not Equal To 0?(x=w253) -> (x != 0?=w248:bool)
                n98 = Select(t=w251, s=w248, f=w250) -> (s? t:f=w252:T13[])
              }
            }
            n99 = call <userlib>:"CalcRate.vi"("Refresh(ms)"=u32 100) -> ("updated?"=w228:bool)  [unwired: 8 in, 2 out]
            n100 = case shown="Vrai" w228 {
              tunnel: w231 -> [_ w241]
              tunnel: w230 -> [_ w240]
              tunnel: [_ MH_UIThread_Cmds."GetAllRates"] -> w229
              frame False {
              }
              frame True {
                n101 = To Double Precision Float(number=w240) -> (double precision float=w245:dbl)
                n102 = To Double Precision Float(number=w241) -> (double precision float=w246:dbl)
                n103 = Power Of 2(x=w246) -> (2^x=w244:dbl)
                n104 = Multiply(x=w244, y=1000.0) -> (x*y=w243:dbl)
                n105 = Divide(x=w243, y=w245) -> (x/y=w247:dbl)
                n106 = local write "DeltaT"(w247) -> ()
              }
            }
            n107 = Build Array (concatenate)(w238, w233, w229) -> (w237:T13[])
          }
          event "BitShift": Value Change {
            n108 = event-data() -> ()  [unwired: 1 in, 1 out]
            n109 = Bundle By Name(cluster=w260, "BitShift"="BitShift") -> (w259:T9)
            n110 = Build Array (concatenate)(w256, MH_UIThread_Cmds."SetBitShift") -> (w255:T13[])
          }
          event "Start": Value Change {
            n111 = event-data() -> ()  [unwired: 1 in, 1 out]
            n112 = Unbundle By Name(w264) -> ("SyncRate"=w263:i32)
            n113 = Greater Or Equal?(x=w263, y=10) -> (x >= y?=w261:bool)
            n114 = case shown="Vrai" w261 {
              selector: w261 -> [w270 _]
              tunnel: w268 -> [w272 w281]
              tunnel: [w272 w279] -> w267
              tunnel: [w271 w278] -> w266
              tunnel: "Start" -> [_ w277]
              tunnel: w264 -> [w271 w273]
              frame False {
                n115 = local write "Start"(w270) -> ()
                n116 = One Button Dialog(message="SyncRate too low!!!" ("Status")) -> ()  [unwired: 1 in, 1 out]
              }
              frame True {
                w276 = T13[] [enum."SetBitShift", enum."SetHistoAcqTime", enum."StartMeas"] items=["Idle", "Init", "SetInpChan", "SetSyncDivider", "SetSyncTrg", "SetSyncOffset", "SetSyncDeadTime", "SetBinning", "SetHistoOffset", "SetHistoLen", "SetStopOvl", "SetBitShift", "SetHistoAcqTime", "GetRates", "GetAllRates", "StartMeas", "StopMeas", "AbortMeas", "GetResolution", "GetHistos", "GetAllHistos", "ReadFiFo", "WriteStatus", "Resize", "EnableControls", "DisableControls", "Error", "Exit"]
                n117 = Bundle By Name(cluster=w273, "StartMeas"=w277) -> (w278:T9)
                n118 = Build Array(MH_UIThread_Cmds."AbortMeas") -> (w274:T13[])
                n119 = Select(t=w276, s=w277, f=w274) -> (s? t:f=w280:T13[])
                n120 = Build Array (concatenate)(w281, w280) -> (w279:T13[])
              }
            }
          }
          event "Run continuously": Value Change {
            n121 = event-data() -> ()  [unwired: 1 in, 1 out]
            n122 = Bundle By Name(cluster=w284, "Run cont."="Run continuously") -> (w283:T9)
          }
          event "Scale": Value Change {
            n123 = event-data() -> ()  [unwired: 1 in, 1 out]
            n124 = Select(t=u8 0 ("Y Scale.Mapping Mode"), s="Scale", f=u8 1 ("Y Scale.Mapping Mode")) -> (s? t:f=w286:u8)
            n125 = property on="HistoGraph" class="GraphWF (strict)"("YScale.Mapping Mode"=w286) -> ()  [unwired: 2 in, 2 out]
          }
          event "Settings": Value Change {
            n126 = event-data() -> ()  [unwired: 1 in, 1 out]
            n127 = property on="Splitter" class="BarreDiv"() -> ("Position"=w297:i32)  [unwired: 2 in, 2 out]
            n128 = Select(t=300 ("PosT"), s="Settings", f=0 ("PosF")) -> (s? t:f=w294:i32)
            n129 = Subtract(x=w297, y=w294) -> (x-y=w293:i32)
            n130 = while {
              shift-right: [w308] -> _
              shift-left: w293 -> [w301]
              i -> [w307]
              stop <- w304 stop-if-true
              n131 = property on="Splitter 4" class="BarreDiv"("Position"=w301) -> (error out=w300:errorcluster)  [unwired: 2 in, 1 out]
              n132 = Greater Or Equal?(x=w307, y=10) -> (x >= y?=w305:bool)
              n133 = Decrement(x=w301) -> (x-1=w308:i32)
              n134 = Unbundle(w300) -> ("status"=w303:bool)  [unwired: 2 out]
              n135 = Not(x=w303) -> (.not. x?=w302:bool)
              n136 = Or(x=w302, y=w305) -> (x .or. y?=w304:bool)
            }
          }
          event Panel Resize {
            n137 = event-data() -> ()  [unwired: 1 in, 1 out]
            n138 = Build Array (concatenate)(w310, MH_UIThread_Cmds."Resize") -> (w309:T13[])
          }
        }
      }
      frame "Init" {
        w324 = 1000 ("SyncDeadTime")
        w325 = FALSE ("UseDeadTime")
        w327 = T17 3 items=["HIST"=0, "T2"=2, "T3"=3]  # Mode
        w329 = MH_RefSource."INTERNAL"  # refsource
        w335 = 1.0 ("HistoAcqTime")
        w336 = 15 ("Value (Signaling)")
        w353 = FALSE ("Run cont.")
        w355 = FALSE ("StartMeas")
        w356 = u32 4294967295 ("OvlLevel")
        w357 = TRUE ("StopOvl.")
        w358 = 360000000 ("AcqTime")
        w359 = 0 ("HistoOffset")
        w360 = 0 ("Binning")
        w361 = -100 ("SyncLevel")
        w362 = 0 ("SyncZeroX")
        w363 = 0 ("SyncOffset")
        w364 = 0 ("SyncDivider")
        w366 = T13[] [enum."SetSyncDivider", enum."SetSyncOffset", enum."SetSyncDeadTime", enum."SetSyncTrg", enum."SetInpChan", enum."SetBinning", enum."SetHistoOffset", enum."Resize", enum."EnableControls", enum."GetRates", enum."SetBitShift", enum."SetHistoAcqTime", enum."WriteStatus"] items=["Idle", "Init", "SetInpChan", "SetSyncDivider", "SetSyncTrg", "SetSyncOffset", "SetSyncDeadTime", "SetBinning", "SetHistoOffset", "SetHistoLen", "SetStopOvl", "SetBitShift", "SetHistoAcqTime", "GetRates", "GetAllRates", "StartMeas", "StopMeas", "AbortMeas", "GetResolution", "GetHistos", "GetAllHistos", "ReadFiFo", "WriteStatus", "Resize", "EnableControls", "DisableControls", "Error", "Exit"]
        # "100 x 60 x 60 x 1000 = 100 h"
        # "Init all FP controls and corresponding copy in UIThread Data cluster"
        # "EnQ list of commands"
        # "Array with Inp.Chan."
        # "Initialization: 1. Init HW -> get # of channels -> make array for Inp.Channels\n2. Init all FP controls and corresponding fields in UIThread Data cluster\n3. EnQ list of commands for further initialization"
        n139 = disable-structure shown="TARGET_TYPE==Windows, Default" {
          disable-tunnel: ["MHLib64" ("name or relative path") "MHLib" ("name or relative path")] -> w326
          frame condition #0 (active) {
          }
          frame condition #1 {
          }
        }
        n140 = call <vilib>:"Error Cluster From Error Code.vi"("is warning? (False)"=FALSE, "show call chain? (False)"=TRUE, "error message (\"\")"="DLL not found!" ("error message (\"\")"), "error code (0)"=5000) -> ("error out"=w330:errorcluster)  [unwired: 5 in]
        n141 = call <userlib>:"MH_GetDLLPath.vi"("DllName_32bit"="MHLib" ("name or relative path"), "DllName_64bit"=w326) -> ("file exists?"=w332:bool, "DLLPath"=w333:path)  [unwired: 8 in]
        n142 = global write "MH_DllPath_global.vi" "DllPath"(w333) -> ()
        n143 = property on="AllChannels" class="Clust (strict)"("Val(Sgnl)"=T1 {"Enable"=TRUE, "Offset"=0, "Level"=-100, "Edge"=0, "DeadTime"=1000, "UseDeadTime"=FALSE, "SetEnableAllChan"=TRUE, "SetEdgeAllChan"=TRUE, "SetLevelAllChan"=TRUE, "SetOffsetAllChan"=TRUE, "SetUseDTAllChan"=TRUE, "SetDeadTAllChan"=TRUE} ("AllChannels")) -> ()  [unwired: 2 in, 2 out]
        n144 = Select(t=errorcluster {"status"=FALSE, "code"=0, "source"=""} ("error IO"), s=w332, f=w330) -> (s? t:f=w347:errorcluster)
        n145 = global read "MH_LibVersion_global.vi" "Library Version"() -> (w328:string)
        n146 = Build Array (concatenate)(w367, w366) -> (w365:T13[])
        n147 = call <userlib>:"InitMH_UIThread.vi"("error in (no error)"=w347, "Mode"=w327, "refsource"=w329, "Library Version"=w328) -> ("error out"=w368:errorcluster, "Init Info"=w370:T10, "DevIdx"=w369:i32)  [unwired: 5 in]
        n148 = local write "SyncDivider"(w364) -> ()
        n149 = local write "SyncOffset"(w363) -> ()
        n150 = local write "SyncEdge"(w362) -> ()
        n151 = local write "SyncLevel"(w361) -> ()
        n152 = local write "Binning"(w360) -> ()
        n153 = Bundle By Name(cluster=w351, "DevIdx"=w369, "Init Info"=w370, "Status"="Initialized!") -> (w350:T9)
        n154 = Unbundle By Name(w350) -> ("Init Info.Bin Steps"=w349:i32, "Init Info.Base Resolution"=w318:dbl, "Init Info.nchannels"=w323:i32)
        n155 = for {
          N: w323 -> [_]
          i -> [w373]
          n156 = Increment(x=w373) -> (x+1=w376:i32)
          n157 = Format Into String(format string="Ch.%d", w376) -> (resulting string=w374:string)  [unwired: 2 in, 1 out]
          n158 = property on="HistoGraph" class="GraphWF (strict)"("Active Plot"=w373, "Plot.Plot Name"=w374) -> ()  [unwired: 2 in, 2 out]
          n159 = property on="TTraceGraph" class="GraphWF (strict)"("Active Plot"=w373, "Plot.Plot Name"=w374) -> ()  [unwired: 2 in, 2 out]
        }
        n160 = Bundle By Name(cluster=T6 {"Histos"=[], "Cmd"=enum."_none_", "TimeTrace"=[], "Bin"=0, "Total bin"=0, "Status"="", "Resol"=0.0, "DeltaT"=0.0, "nChannels"=0} ("MH_GUIThread_QData"), "Cmd"=MH_VisThread_QCmds."nChannels", "nChannels"=w323) -> (w339:T6)
        n161 = To Unsigned Long Integer(number=w318) -> (unsigned 32bit integer=w319:u32)
        n162 = property on="Offset" class="NumNb (strict)"("Increment"=w318) -> ()  [unwired: 2 in, 2 out]
        n163 = property on="SyncOffset" class="NumNb (strict)"("Increment"=w318) -> ()  [unwired: 2 in, 2 out]
        n164 = property on="Offset" class="NumNb (strict)"("Increment"=w318) -> ()  [unwired: 2 in, 2 out]
        n165 = Bundle By Name(cluster=T8 {"Cmd"=enum."Proc", "nActual"=0, "Buffer"=[], "TickCount"=0, "Param"=0} ("MH_DataProcThread_QData"), "Param"=w323, "Cmd"=MH_DataProcThread_QCmds."SetNumChannels") -> (w343:T8)
        n166 = call <userlib>:"MH_CalcBinningValues.vi"("BaseResolution"=w319, "Bin Steps"=w349) -> ("BinningValues"=w354:cluster{"String":string, "Value":i32}[])  [unwired: 9 in]
        n167 = Enqueue Element(queue=w337, element=w339) -> ()  [unwired: 2 in, 3 out]
        n168 = property on="Binning" class="MDér (strict)"("StringsAndValues[]"=w354) -> ()  [unwired: 2 in, 2 out]
        n169 = Enqueue Element(queue=w344, element=w343) -> ()  [unwired: 2 in, 3 out]
        n170 = call <userlib>:"MH_InitChannels.vi"("nchannels"=w323) -> ("SetInpChan"=w321:T11[], "Channels"=w322:T3[])  [unwired: 9 in]
        n171 = local write "Channels"(w322) -> ()
        n172 = Bundle By Name(cluster=w350, "Channels"=w322, "SetInpChan"=w321, "SyncDivider"=w364, "SyncOffset"=w363, "SyncEdge"=w362, "SyncLevel"=w361, "Binning"=w360, "HistoOffset"=w359, "AcqTime"=w358, "StopOvl."=w357, "OvlLevel"=w356, "StartMeas"=w355, "Run cont."=w353, "BitShift"=w336, "HistoAcqTime"=w335, "UseDeadTime"=w325, "SyncDeadTime"=w324) -> (w346:T9)
        n173 = local write "StopOvl."(w357) -> ()
        n174 = local write "OvlLevel"(w356) -> ()
        n175 = local write "Start"(w355) -> ()
        n176 = local write "Run continuously"(w353) -> ()
        n177 = local write "BitShift"(w336) -> ()
        n178 = local write "HistoOffset"(w359) -> ()
        n179 = local write "AcqTime"(w358) -> ()
        n180 = local write "HistoAcqTime"(w335) -> ()
        n181 = local write "UseDeadTime"(w325) -> ()
        n182 = local write "SyncDeadTime"(w324) -> ()
        n183 = property on="Settings" class="Bool (strict)"("Val(Sgnl)"=TRUE ("Value (Signaling)")) -> ()  [unwired: 2 in, 2 out]
        n184 = property on="Scale" class="Bool (strict)"("Val(Sgnl)"=FALSE ("Value (Signaling)")) -> ()  [unwired: 2 in, 2 out]
      }
      frame "SetInpChan" {
        n185 = Unbundle By Name(w385) -> ("DevIdx"=w383:i32, "Init Info.features"=w382:i32, "SetInpChan"=w381:T11[], "Channels"=w380:T3[])
        n186 = for {
          tunnel: w380 -> [w390]
          tunnel: w381 -> [w394] mode=indexing
          shift-right: [w392] -> w379
          shift-left: errorcluster {"status"=FALSE, "code"=0, "source"=""} ("error out") -> [w391]
          tunnel: w383 -> [w388]
          tunnel: w382 -> [w386]
          n187 = Unbundle By Name(w394) -> ("Cmds"=w393:T12[], "Channel"=w387:i32)
          n188 = Index Array(array=w390, index=w387) -> (element=w389:T3)
          n189 = for {
            tunnel: w393 -> [w401] mode=indexing
            tunnel: w387 -> [w400]
            shift-right: [w399] -> w392
            shift-left: w391 -> [w398]
            tunnel: w389 -> [w397]
            tunnel: w388 -> [w396]
            tunnel: w386 -> [w395]
            n190 = case shown="\"SetInpChanDeadTime\"" w401 {
              tunnel: w400 -> [_ w407 w414 w419 w435]
              tunnel: [w402 w406 w413 w423 w440] -> w399
              tunnel: w398 -> [w402 w405 w412 w422 w439]
              tunnel: w397 -> [_ w404 w411 w421 w438]
              tunnel: w396 -> [_ w403 w410 w420 w437]
              tunnel: w395 -> [_ _ _ w416 _]
              frame Default {
              }
              frame "SetInpChanEnable" {
                n191 = Unbundle By Name(w404) -> ("Enable"=w408:bool)
                n192 = call <userlib>:"MH_SetInputChannelEnable.vi"("error in (no error)"=w405, "enable"=w408, "channel"=w407, "devidx"=w403) -> ("error out"=w406:errorcluster)  [unwired: 6 in, 1 out]
              }
              frame "SetInpChanOffset" {
                n193 = Unbundle By Name(w411) -> ("Offset"=w409:i32)
                n194 = call <userlib>:"MH_SetInputChannelOffset.vi"("error in (no error)"=w412, "Offset"=w409, "channel"=w414, "devidx"=w410) -> ("error out"=w413:errorcluster)  [unwired: 6 in, 1 out]
              }
              frame "SetInpChanDeadTime" {
                w417 = 32  # FEATURE_PROG_TD
                n195 = And(x=w416, y=w417) -> (x .and. y?=w418:i32)
                n196 = Not Equal To 0?(x=w418) -> (x != 0?=w415:bool)
                n197 = case shown="Faux" w415 {
                  tunnel: [w424 w433] -> w423
                  tunnel: w422 -> [w424 w432]
                  tunnel: w421 -> [_ w431]
                  tunnel: w420 -> [_ w430]
                  tunnel: w419 -> [_ w428]
                  frame False {
                  }
                  frame True {
                    n198 = Unbundle By Name(w431) -> ("UseDeadTime"=w427:bool, "DeadTime"=w429:i32)
                    n199 = Boolean To (0,1)(Boolean=w427) -> (0, 1=w426:i16)
                    n200 = To Long Integer(number=w426) -> (32bit integer=w425:i32)
                    n201 = call <userlib>:"MH_SetInputDeadTime.vi"("channel"=w428, "error in (no error)"=w432, "deadtime"=w429, "on"=w425, "devidx"=w430) -> ("error out"=w433:errorcluster)  [unwired: 5 in, 1 out]
                  }
                }
              }
              frame "SetInpChanTrg" {
                n202 = Unbundle By Name(w438) -> ("Level"=w434:i32, "Edge"=w436:i32)
                n203 = call <userlib>:"MH_SetInputEdgeTrg.vi"("channel"=w435, "error in (no error)"=w439, "edge"=w436, "level"=w434, "devidx"=w437) -> ("error out"=w440:errorcluster)  [unwired: 5 in, 1 out]
              }
            }
          }
        }
      }
      frame "SetSyncDivider" {
        n204 = Unbundle By Name(w449) -> ("DevIdx"=w448:i32, "SyncDivider"=w444:i32)
        n205 = Power Of 2(x=w444) -> (2^x=w443:dbl)
        n206 = To Long Integer(number=w443) -> (32bit integer=w442:i32)
        n207 = call <userlib>:"MH_SetSyncDiv.vi"("SyncDivider"=w442, "devidx"=w448) -> ("error out"=w446:errorcluster)  [unwired: 8 in, 1 out]
        n208 = flat-sequence {
          tunnel: w446 -> [w450]
          tunnel: [w450] -> w445
          frame #0 {
            n209 = Wait (ms)(milliseconds to wait=u32 100) -> ()  [unwired: 1 out]
          }
        }
      }
      frame "SetSyncTrg" {
        n210 = Unbundle By Name(w458) -> ("DevIdx"=w455:i32, "SyncLevel"=w453:i32, "SyncEdge"=w454:i32)
        n211 = call <userlib>:"MH_SetSyncEdgeTrg.vi"("edge"=w454, "level"=w453, "devidx"=w455) -> ("error out"=w456:errorcluster)  [unwired: 7 in, 1 out]
      }
      frame "SetSyncDeadTime" {
        w462 = 32  # FEATURE_PROG_TD
        n212 = Unbundle By Name(w471) -> ("DevIdx"=w468:i32, "UseDeadTime"=w465:bool, "SyncDeadTime"=w467:i32, "Init Info.features"=w461:i32)
        n213 = And(x=w461, y=w462) -> (x .and. y?=w463:i32)
        n214 = Boolean To (0,1)(Boolean=w465) -> (0, 1=w466:i16)
        n215 = Not Equal To 0?(x=w463) -> (x != 0?=w460:bool)
        n216 = To Long Integer(number=w466) -> (32bit integer=w464:i32)
        n217 = case shown="Vrai" w460 {
          tunnel: [_ w475] -> w469
          tunnel: w468 -> [_ w474]
          tunnel: w467 -> [_ w473]
          tunnel: w464 -> [_ w472]
          frame False {
          }
          frame True {
            n218 = call <userlib>:"MH_SetSyncDeadTime.vi"("deadtime"=w473, "on"=w472, "devidx"=w474) -> ("error out"=w475:errorcluster)  [unwired: 7 in, 1 out]
          }
        }
      }
      frame "SetSyncOffset" {
        n219 = Unbundle By Name(w481) -> ("DevIdx"=w479:i32, "SyncOffset"=w478:i32)
        n220 = call <userlib>:"MH_SetSyncChannelOffset.vi"("Offset"=w478, "devidx"=w479) -> ("error out"=w480:errorcluster)  [unwired: 8 in, 1 out]
      }
      frame "SetBinning" {
        # "When binning is changed the new resolution is querried"
        n221 = Unbundle By Name(w489) -> ("DevIdx"=w487:i32, "Binning"=w486:i32)
        n222 = call <userlib>:"MH_SetBinning.vi"("Binning"=w486, "devidx"=w487) -> ("error out"=w488:errorcluster)  [unwired: 8 in, 1 out]
        n223 = Build Array (concatenate)(MH_UIThread_Cmds."GetResolution", w484) -> (w485:T13[])
      }
      frame "SetHistoOffset" {
        n224 = Unbundle By Name(w495) -> ("DevIdx"=w492:i32, "HistoOffset"=w491:i32)
        n225 = call <userlib>:"MH_SetOffset.vi"("Offset"=w491, "devidx"=w492) -> ("error out"=w493:errorcluster)  [unwired: 8 in, 1 out]
      }
      frame "SetStopOvl" {
        n226 = Unbundle By Name(w503) -> ("DevIdx"=w500:i32, "StopOvl."=w499:bool, "OvlLevel"=w498:u32)
        n227 = To Unsigned Long Integer(number=w498) -> (unsigned 32bit integer=w497:u32)
        n228 = call <userlib>:"MH_SetStopOverflow.vi"("stopcount"=w497, "StopOnOverflow"=w499, "devidx"=w500) -> ("error out"=w501:errorcluster)  [unwired: 7 in, 1 out]
      }
      frame "SetBitShift" {
        n229 = Unbundle By Name(w508) -> ("BitShift"=w506:i32, "SyncRate"=w507:i32)
        n230 = Negate(x=w506) -> (-x=w516:i32)
        n231 = Bundle By Name(cluster=T8 {"Cmd"=enum."Proc", "nActual"=0, "Buffer"=[], "TickCount"=0, "Param"=0} ("MH_DataProcThread_QData"), "Param"=w516, "Cmd"=MH_DataProcThread_QCmds."SetShift") -> (w522:T8)
        n232 = To Double Precision Float(number=w506) -> (double precision float=w521:dbl)
        n233 = To Double Precision Float(number=w507) -> (double precision float=w520:dbl)
        n234 = Power Of 2(x=w521) -> (2^x=w519:dbl)
        n235 = Enqueue Element(queue=w509, element=w522) -> ()  [unwired: 2 in, 3 out]
        n236 = Multiply(x=w519, y=1000.0) -> (x*y=w518:dbl)
        n237 = Divide(x=w518, y=w520) -> (x/y=w505:dbl)
        "DeltaT" <- w505
        n238 = Bundle By Name(cluster=T6 {"Histos"=[], "Cmd"=enum."_none_", "TimeTrace"=[], "Bin"=0, "Total bin"=0, "Status"="", "Resol"=0.0, "DeltaT"=0.0, "nChannels"=0} ("MH_GUIThread_QData"), "DeltaT"=w505, "Cmd"=MH_VisThread_QCmds."DeltaT") -> (w517:T6)
        n239 = Enqueue Element(queue=w510, element=w517) -> ()  [unwired: 2 in, 3 out]
      }
      frame "SetHistoAcqTime" {
        n240 = Unbundle By Name(w526) -> ("SyncRate"=w532:i32, "HistoAcqTime"=w525:dbl)
        n241 = To Double Precision Float(number=w532) -> (double precision float=w535:dbl)
        n242 = Multiply(x=w535, y=w525) -> (x*y=w534:dbl)
        n243 = Round To Nearest(number=w534) -> (nearest integer value=w533:dbl)
        n244 = To Long Integer(number=w533) -> (32bit integer=w531:i32)
        n245 = Bundle By Name(cluster=T8 {"Cmd"=enum."Proc", "nActual"=0, "Buffer"=[], "TickCount"=0, "Param"=0} ("MH_DataProcThread_QData"), "Param"=w531, "Cmd"=MH_DataProcThread_QCmds."SetHistAcqTime") -> (w530:T8)
        n246 = Enqueue Element(queue=w527, element=w530) -> ()  [unwired: 2 in, 3 out]
      }
      frame "GetAllRates" {
        # "An alternative to GetRates"
        n247 = Unbundle By Name(w539) -> ("DevIdx"=w547:i32, "Init Info.nchannels"=w554:i32, "StartMeas"=w548:bool, "SyncRateStart"=w542:i32)
        n248 = call <userlib>:"MH_AllocateCntRateBuffer.vi"("NumChan"=w554) -> ("Buffer"=w553:i32[])  [unwired: 10 in]
        n249 = call <userlib>:"MH_GetAllCountRates.vi"("cntrates_buf"=w553, "devidx"=w547) -> ("error out"=w546:errorcluster, "cntrates"=→"CountRates":i32[], "syncrate"=w544:i32)  [unwired: 6 in, 1 out]
        n250 = case shown="Vrai" w548 {
          tunnel: w547 -> [_ w569]
          tunnel: w546 -> [w558 w568]
          tunnel: [w558 w567] -> w545
          tunnel: w544 -> [w557 _]
          tunnel: [w557 w564] -> w543
          tunnel: w542 -> [_ w559]
          tunnel: w541 -> [w556 w563]
          tunnel: [w556 w562] -> w540
          tunnel: w539 -> [w555 w561]
          tunnel: [w555 w560] -> w538
          frame False {
          }
          frame True {
            n251 = call <userlib>:"MH_GetSyncPeriod.vi"("error in (no error)"=w568, "devidx"=w569) -> ("error out"=w567:errorcluster, "period"=w566:dbl)  [unwired: 7 in, 1 out]
            n252 = Reciprocal(x=w566) -> (1/x=w565:dbl)
            n253 = To Long Integer(number=w565) -> (32bit integer=w564:i32)
            n254 = case shown="Par défaut" w559 {
              selector: w559 -> [w570 _ _]
              tunnel: w564 -> [w573 w594 _]
              tunnel: w563 -> [w571 w596 w600]
              tunnel: [w572 w596 w600] -> w562
              tunnel: w561 -> [w577 w595 w599]
              tunnel: [w577 w593 w598] -> w560
              frame Default {
                n255 = Subtract(x=w573, y=w570) -> (x-y=w576:i32)
                n256 = Absolute Value(x=w576) -> (abs(x)=w574:i32)
                n257 = Not Equal To 0?(x=w574) -> (x != 0?=w575:bool)
                n258 = case shown="Vrai" w575 {
                  tunnel: w574 -> [_ w586]
                  tunnel: [w578 w581] -> w572
                  tunnel: w571 -> [w578 w580]
                  tunnel: w570 -> [_ w579]
                  frame False {
                  }
                  frame True {
                    n259 = To Double Precision Float(number=w586) -> (double precision float=w585:dbl)
                    n260 = To Double Precision Float(number=w579) -> (double precision float=w587:dbl)
                    n261 = Divide(x=w585, y=w587) -> (x/y=w584:dbl)
                    n262 = Greater Or Equal?(x=w584, y=0.01) -> (x >= y?=w582:bool)
                    n263 = case shown="Vrai" w582 {
                      tunnel: [w588 w591] -> w581
                      tunnel: w580 -> [w588 w589]
                      frame False {
                      }
                      frame True {
                        w590 = T13[] [enum."StopMeas"] items=["Idle", "Init", "SetInpChan", "SetSyncDivider", "SetSyncTrg", "SetSyncOffset", "SetSyncDeadTime", "SetBinning", "SetHistoOffset", "SetHistoLen", "SetStopOvl", "SetBitShift", "SetHistoAcqTime", "GetRates", "GetAllRates", "StartMeas", "StopMeas", "AbortMeas", "GetResolution", "GetHistos", "GetAllHistos", "ReadFiFo", "WriteStatus", "Resize", "EnableControls", "DisableControls", "Error", "Exit"]
                        n264 = One Button Dialog(message="Warning: Sync Rate has changed!\nTime Trace resolution has been changed accordingly.\nMeasurement is aborted.\n") -> ()  [unwired: 1 in, 1 out]
                        n265 = Build Array (concatenate)(w589, w590) -> (w591:T13[])
                      }
                    }
                  }
                }
              }
              frame -1 {
                n266 = Bundle By Name(cluster=w595, "SyncRateStart"=w594) -> (w593:T9)
              }
              frame -2 {
                n267 = Bundle By Name(cluster=w599, "SyncRateStart"=-1) -> (w598:T9)
              }
            }
          }
        }
        n268 = Bundle By Name(cluster=w538, "SyncRate"=w543) -> (w549:T9)
        n269 = Format Into String(format string="Sync Rate: %d cps\n", w543) -> (resulting string=→"SyncRate":string)  [unwired: 2 in, 1 out]
      }
      frame "GetRates" {
        # "An alternative to GetAllRates"
        n270 = Unbundle By Name(w606) -> ("Init Info.nchannels"=w611:i32, "Channels"=w607:T3[], "DevIdx"=w608:i32)
        n271 = call <userlib>:"MH_GetSyncRate.vi"("devidx"=w608) -> ("error out"=w610:errorcluster, "syncrate"=w604:i32)  [unwired: 8 in, 1 out]
        n272 = Format Into String(format string="Sync Rate: %d cps\n", w604) -> (resulting string=w603:string)  [unwired: 2 in, 1 out]
        n273 = local write "SyncRate"(w603) -> ()
        n274 = for {
          N: w611 -> [_]
          tunnel: w608 -> [w619]
          tunnel: [w616] -> w602 mode=indexing
          shift-right: [w618] -> w612
          shift-left: w610 -> [w620]
          tunnel: w607 -> [w615] mode=indexing
          i -> [w617]
          n275 = Unbundle By Name(w615) -> ("Enable"=w614:bool)
          n276 = case shown="Vrai" w614 {
            tunnel: w620 -> [w621 w626]
            tunnel: w619 -> [_ w625]
            tunnel: [w621 w624] -> w618
            tunnel: w617 -> [_ w623]
            tunnel: [_ w622] -> w616
            frame False {
            }
            frame True {
              n277 = call <userlib>:"MH_GetCountRate.vi"("error in (no error)"=w626, "Channel"=w623, "devidx"=w625) -> ("error out"=w624:errorcluster, "rate"=w622:i32)  [unwired: 6 in, 1 out]
            }
          }
        }
        n278 = local write "CountRates"(w602) -> ()
        n279 = Bundle By Name(cluster=w606, "SyncRate"=w604) -> (w605:T9)
      }
      frame "StartMeas" {
        n280 = Bundle By Name(cluster=T8 {"Cmd"=enum."Proc", "nActual"=0, "Buffer"=[], "TickCount"=0, "Param"=0} ("MH_DataProcThread_QData"), "Cmd"=MH_DataProcThread_QCmds."Init") -> (w632:T8)
        n281 = Unbundle By Name(w630) -> ("DevIdx"=w639:i32, "AcqTime"=w635:i32)
        n282 = Enqueue Element(queue=w634, element=w632) -> ()  [unwired: 2 in, 3 out]
        n283 = Bundle By Name(cluster=w630, "SyncRateStart"=-2) -> (w629:T9)
        n284 = call <userlib>:"MH_StartMeas.vi"("tacq"=w635, "devidx"=w639) -> ("error out"=w640:errorcluster)  [unwired: 8 in, 1 out]
        n285 = Build Array (concatenate)(w638, MH_UIThread_Cmds."ReadFiFo") -> (w637:T13[])
      }
      frame "StopMeas" {
        n286 = Unbundle By Name(w647) -> ("Run cont."=w642:bool, "DevIdx"=w648:i32)
        n287 = call <userlib>:"MH_StopMeas.vi"("devidx"=w648) -> ("error out"=w649:errorcluster)  [unwired: 9 in, 1 out]
        n288 = case shown="Faux" w642 {
          tunnel: w647 -> [w653 w655]
          tunnel: [w652 w655] -> w646
          tunnel: [w650 w654] -> w645
          frame False {
            w650 = T13[] [enum."ReadFiFo"] items=["Idle", "Init", "SetInpChan", "SetSyncDivider", "SetSyncTrg", "SetSyncOffset", "SetSyncDeadTime", "SetBinning", "SetHistoOffset", "SetHistoLen", "SetStopOvl", "SetBitShift", "SetHistoAcqTime", "GetRates", "GetAllRates", "StartMeas", "StopMeas", "AbortMeas", "GetResolution", "GetHistos", "GetAllHistos", "ReadFiFo", "WriteStatus", "Resize", "EnableControls", "DisableControls", "Error", "Exit"]
            w651 = FALSE ("StartMeas")
            n289 = Bundle By Name(cluster=w653, "StartMeas"=w651) -> (w652:T9)
            n290 = local write "Start"(w651) -> ()
          }
          frame True {
            w654 = T13[] [enum."ReadFiFo", enum."StartMeas"] items=["Idle", "Init", "SetInpChan", "SetSyncDivider", "SetSyncTrg", "SetSyncOffset", "SetSyncDeadTime", "SetBinning", "SetHistoOffset", "SetHistoLen", "SetStopOvl", "SetBitShift", "SetHistoAcqTime", "GetRates", "GetAllRates", "StartMeas", "StopMeas", "AbortMeas", "GetResolution", "GetHistos", "GetAllHistos", "ReadFiFo", "WriteStatus", "Resize", "EnableControls", "DisableControls", "Error", "Exit"]
          }
        }
        n291 = Build Array (concatenate)(w644, w645) -> (w643:T13[])
      }
      frame "AbortMeas" {
        w658 = FALSE ("StartMeas")
        n292 = Unbundle By Name(w660) -> ("DevIdx"=w661:i32)
        n293 = call <userlib>:"MH_StopMeas.vi"("devidx"=w661) -> ("error out"=w662:errorcluster)  [unwired: 9 in, 1 out]
        n294 = Bundle By Name(cluster=w660, "StartMeas"=w658) -> (w659:T9)
        n295 = local write "Start"(w658) -> ()
      }
      frame "GetResolution" {
        # "Resolution in ns"
        # "Gets resolution in ps"
        # "Resolution is saved in UIThread Data cluster in ns"
        n296 = Unbundle By Name(w672) -> ("DevIdx"=w674:i32)
        n297 = call <userlib>:"MH_GetResolution.vi"("devidx"=w674) -> ("error out"=w673:errorcluster, "resolution"=w670:dbl)  [unwired: 8 in, 1 out]
        n298 = Divide(x=w670, y=1000.0) -> (x/y=w666:dbl)
        n299 = Bundle By Name(cluster=w672, "Resolution"=w666) -> (w671:T9)
        n300 = Bundle By Name(cluster=T6 {"Histos"=[], "Cmd"=enum."_none_", "TimeTrace"=[], "Bin"=0, "Total bin"=0, "Status"="", "Resol"=0.0, "DeltaT"=0.0, "nChannels"=0} ("MH_GUIThread_QData"), "Resol"=w666, "Cmd"=MH_VisThread_QCmds."Resol") -> (w664:T6)
        n301 = Enqueue Element(queue=w668, element=w664) -> ()  [unwired: 2 in, 3 out]
      }
      frame "ReadFiFo" {
        w686 = 2  # FLAG_FIFOFULL
        # "Reads photon records from HW and transferes them to DataProcThread via Queue."
        n302 = Unbundle By Name(w688) -> ("DevIdx"=w682:i32)
        n303 = call <userlib>:"MH_GetFlags.vi"("devidx"=w682) -> ("error out"=w684:errorcluster, "flags"=w685:i32)  [unwired: 8 in, 1 out]
        n304 = And(x=w685, y=w686) -> (x .and. y?=w687:i32)
        n305 = Not Equal To 0?(x=w687) -> (x != 0?=w681:bool)
        "OverRun" <- w681
        n306 = case shown="Faux" w681 {
          tunnel: w684 -> [w700 w704]
          tunnel: [w699 w704] -> w683
          tunnel: w682 -> [w692 _]
          tunnel: w680 -> [w698 _]
          tunnel: w679 -> [w697 _]
          tunnel: [w697 w702] -> w678
          tunnel: w677 -> [w690 w701]
          tunnel: [w689 w701] -> w676
          frame False {
            n307 = call <userlib>:"MH_ReadFiFo.vi"("error in (no error)"=w700, "devidx"=w692) -> ("error out"=w699:errorcluster, "nactual"=w691:i32, "buffer"=w695:u32[])  [unwired: 6 in, 1 out]
            n308 = Bundle By Name(cluster=T8 {"Cmd"=enum."Proc", "nActual"=0, "Buffer"=[], "TickCount"=0, "Param"=0} ("MH_DataProcThread_QData"), "Buffer"=w695, "nActual"=w691, "Cmd"=MH_DataProcThread_QCmds."Proc") -> (w693:T8)
            n309 = Increment(x=w690) -> (x+1=w689:i32)
            n310 = Enqueue Element(queue=w698, element=w693) -> ()  [unwired: 2 in, 3 out]
          }
          frame True {
            n311 = Build Array(MH_UIThread_Cmds."AbortMeas") -> (w702:T13[])
          }
        }
      }
      frame "WriteStatus" {
        n312 = Unbundle By Name(w707) -> ("Status"=→"Status":string)
      }
      frame "Resize" {
        n313 = property on="Pane 3" class="Pann"() -> ("Width"=w715:u32)  [unwired: 2 in, 2 out]
        n314 = Subtract(x=w715, y=i16 100 ("b")) -> (x-y=w721:u32)
        n315 = Unbundle By Name(w710) -> ("Init Info.nchannels"=w718:i32)
        n316 = Quotient & Remainder(x=w721, y=i16 99 ("m")) -> (floor(x/y)=w720:u32)  [unwired: 1 out]
        n317 = In Range and Coerce(upper limit=w718, x=w720, lower limit=4) -> (coerced(x)=w719:u32)  [unwired: 1 out]
        n318 = Equal?(x=w718, y=w719) -> (x = y?=w717:bool)
        n319 = Not(x=w717) -> (.not. x?=w716:bool)
        n320 = property on="Channels" class="Tabl (strict)"("HorizScroll"=w716, "Number of Columns"=w719, "Index Values"=u32[] [0]) -> ()  [unwired: 2 in, 2 out]
      }
      frame "EnableControls" {
        n321 = property class="VI"() -> ("Panel"=w727:refnum<vi>)  [unwired: 2 in, 2 out]
        n322 = property class="FA"(reference=w727) -> ("Decos[]"=w728:refnum<vi>[])  [unwired: 1 in, 2 out]
        n323 = property class="FA"(reference=w727) -> ("Controls[]"=w726:refnum<vi>[])  [unwired: 1 in, 2 out]
        n324 = for {
          tunnel: w728 -> [w732] mode=indexing
          tunnel: TRUE -> [w731]
          n325 = property class="Déco"(reference=w732, "Visible"=w731) -> ()  [unwired: 1 in, 2 out]
        }
        n326 = for {
          tunnel: w726 -> [w735] mode=indexing
          tunnel: T14."Enabled" ("Disabled") -> [w734]
          tunnel: [w733] -> _
          n327 = property class="Cmde"(reference=w735, "DisabledEnum"=w734) -> (error out=w733:errorcluster)  [unwired: 1 in, 1 out]
        }
      }
      frame "DisableControls" {
        n328 = property class="VI"() -> ("Panel"=w740:refnum<vi>)  [unwired: 2 in, 2 out]
        n329 = property class="FA"(reference=w740) -> ("Decos[]"=w741:refnum<vi>[])  [unwired: 1 in, 2 out]
        n330 = property class="FA"(reference=w740) -> ("Controls[]"=w739:refnum<vi>[])  [unwired: 1 in, 2 out]
        n331 = for {
          tunnel: w741 -> [w745] mode=indexing
          tunnel: FALSE -> [w744]
          n332 = property class="Déco"(reference=w745, "Visible"=w744) -> ()  [unwired: 1 in, 2 out]
        }
        n333 = for {
          tunnel: w739 -> [w748] mode=indexing
          tunnel: T14."Disabled and Grayed Out" ("Disabled") -> [w747]
          tunnel: [w746] -> _
          n334 = property class="Cmde"(reference=w748, "DisabledEnum"=w747) -> (error out=w746:errorcluster)  [unwired: 1 in, 1 out]
        }
      }
      frame "Error" {
        w750 = T13[] [enum."Exit"] items=["Idle", "Init", "SetInpChan", "SetSyncDivider", "SetSyncTrg", "SetSyncOffset", "SetSyncDeadTime", "SetBinning", "SetHistoOffset", "SetHistoLen", "SetStopOvl", "SetBitShift", "SetHistoAcqTime", "GetRates", "GetAllRates", "StartMeas", "StopMeas", "AbortMeas", "GetResolution", "GetHistos", "GetAllHistos", "ReadFiFo", "WriteStatus", "Resize", "EnableControls", "DisableControls", "Error", "Exit"]
        w753 = T19 1 items=["no dialog", "OK message", "continue or stop message", "OK message + warnings", "continue/stop + warnings"] ("type of dialog (OK msg:1)")
        # "Error case: If an error occures the user is informed and the programm terminates. Add your own code to handle error events (e.g. exception lists, etc.)"
        n335 = call <vilib>:"Simple Error Handler.vi"("type of dialog (OK msg:1)"=w753, "error in (no error)"=w752) -> ()  [unwired: 3 in, 5 out]
      }
      frame "Exit" {
        n336 = Release Queue(queue=w756) -> ()  [unwired: 2 in, 3 out]
        n337 = Release Queue(queue=w755) -> ()  [unwired: 2 in, 3 out]
        n338 = Unbundle By Name(w760) -> ("DevIdx"=w759:i32)
        n339 = call <userlib>:"MH_CloseDevice.vi"("devidx"=w759) -> ("error out"=w758:errorcluster)  [unwired: 9 in, 1 out]
      }
    }
    n340 = call <userlib>:"MH_EnQError.vi"("error in (no error)"=w28, "Cmds_in"=w26) -> ("error out"=w27:errorcluster, "Cmds_out"=w25:T13[])  [unwired: 8 in]
  }
  n341 = call <userlib>:"MH_DataProcThread.vi"("MH_VisThread_QRef"=w8, "MH_DataProcThread_QRef"=w2) -> ()  [unwired: 10 in]
  n342 = while {
    tunnel: w8 -> [w769]
    shift-right: [w765] -> _
    shift-left: T5 {"Resol"=0.0, "DeltaT"=0.0, "NumChannels"=0} -> [w766]
    tunnel: w2 -> [w764]
    stop <- w762 stop-if-true
    # "VisualizationThread"
    n343 = Dequeue Element(queue=w769, timeout in ms (-1)=100) -> (element=w767:T6, error out=w762:errorcluster)  [unwired: 1 in, 2 out]
    n344 = Unbundle By Name(w767) -> ("Cmd"=w768:T7)
    n345 = case shown="\"Histo\"" w768 {
      tunnel: w767 -> [_ w782 w784 w796 w804 w808 w812]
      tunnel: w766 -> [w772 w780 w786 w788 w803 w807 w811]
      tunnel: [w772 w780 w785 w788 w803 w806 w810] -> w765
      tunnel: w764 -> [w771 _ _ _ w800 _ _]
      tunnel: w762 -> [w770 _ _ _ _ _ _]
      frame "_none_", Default {
        n346 = case shown="Pas d'erreur" w770 {
          tunnel: w771 -> [w776 _]
          frame No Error {
            n347 = Get Queue Status(queue=w776) -> (# elements in queue=w774:i32)  [unwired: 2 in, 7 out]
            n348 = Format Into String(format string="Elements in Q: %d", w774) -> (resulting string=w773:string)  [unwired: 2 in, 1 out]
            n349 = local write "Status"(w773) -> ()
          }
          frame Error {
          }
        }
      }
      frame "Histo" {
        n350 = Unbundle By Name(w782) -> ("Histos"=w777:u32[][])
        n351 = Unbundle By Name(w780) -> ("Resol"=w779:dbl)
        n352 = Bundle(0.0, "Resol"=w779, "Histos"=w777) -> (→"HistoGraph":cluster{dbl, "Resol":dbl, "Histos":u32[][]})  [unwired: 1 in]
      }
      frame "nChannels" {
        n353 = Unbundle By Name(w784) -> ("nChannels"=w783:i32)
        n354 = Bundle By Name(cluster=w786, "NumChannels"=w783) -> (w785:T5)
      }
      frame "TTrace" {
        n355 = Unbundle By Name(w796) -> ("Total bin"=w795:u64, "Bin"=w794:i32, "TimeTrace"=w793:u32[][])
        n356 = Unbundle By Name(w788) -> ("DeltaT"=w787:dbl)
        n357 = call <userlib>:"MH_TTraceToGraph.vi"("DeltaT"=w787, "TimeTrace"=w793, "Bin"=w794, "Total bin"=w795) -> ("TimeTrace_out"=w790:u32[][], "dt"=w791:dbl, "T0"=w792:dbl)  [unwired: 5 in]
        n358 = Bundle("T0"=w792, "dt"=w791, "TimeTrace_out"=w790) -> (→"TTraceGraph":T20)  [unwired: 1 in]
      }
      frame "Status" {
        n359 = Unbundle By Name(w804) -> ("Status"=w801:string)
        n360 = Get Queue Status(queue=w800) -> (# elements in queue=w799:i32)  [unwired: 2 in, 7 out]
        n361 = Format Into String(format string="\t\tElements in Q: %d", w799) -> (resulting string=w797:string)  [unwired: 2 in, 1 out]
        n362 = Concatenate Strings(w801, w797) -> (w802:string)
        n363 = local write "Status"(w802) -> ()
      }
      frame "DeltaT" {
        n364 = Unbundle By Name(w808) -> ("DeltaT"=w805:dbl)
        n365 = Bundle By Name(cluster=w807, "DeltaT"=w805) -> (w806:T5)
      }
      frame "Resol" {
        n366 = Unbundle By Name(w812) -> ("Resol"=w809:dbl)
        n367 = Bundle By Name(cluster=w811, "Resol"=w809) -> (w810:T5)
      }
    }
  }
